vi "QuantelDataGrab.vi"(9 "stop":bool) -> ()   [LabVIEW 2022 SP3]
uses:
  ScanningControl/Pulsers/pulser.ctl
  ScanningControl/Pulsers/UTEX/Controls/UTEX Controls.ctl
  <vilib>/Utility/miscctls.llb/LVRectTypeDef.ctl
  <vilib>/Utility/miscctls.llb/LVBoundsTypeDef.ctl
  ScanningControl/Motion Controllers/NI_controller/-NI_MotionRoutines/MotionParameters.ctl
  ScanningControl/Motion Controllers/NI_controller/-NI_MotionRoutines/MotionSys.ctl
  ScanningControl/Motion Controllers/-MotionRoutines/ScanAxis.ctl
  ScanningControl/Motion Controllers/-MotionRoutines/3rdAxis.ctl
  <vilib>/Utility/miscctls.llb/LVCursorListTypeDef.ctl
  ScanningControl/-ScanSystem/Controls/location.ctl
  ScanningControl/Digitizers/-DigitizerRoutines/Digitizer.ctl
  <vilib>/picture/picture.llb/imagedata.ctl
  <vilib>/Platform/TimedLoop/XDataNode/timing_clust.ctl
  <vilib>/Platform/TimedLoop/XDataNode/nitl_modes.ctl
  <vilib>/Platform/TimedLoop/XDataNode/wakeup.ctl
  <vilib>/event_ctls.llb/eventvkey.ctl
  <vilib>/DAQmx/write.llb/DAQmx Write (Digital Bool 1Line 1Point).vi
  <vilib>/Utility/error.llb/Trim Whitespace One-Sided.vi
  ScanningControl/Pulsers/PulserGlobals.vi
  ScanningControl/Digitizers/-DigitizerRoutines/DigitizerGlobals.vi
  ScanningControl/Motion Controllers/-MotionRoutines/MotionGlobals.vi
  <vilib>/DAQmx/miscellaneous.llb/DAQmx Fill In Error Info.vi
  C:/Windows/System32/ADQAPI_dotNet_helper.dll
  Windows/System32/ADQAPI_dotNet_helper.dll
  <vilib>/Platform/TimedLoop/XDataNode/XDataNode.xnode
  <instrlib>/Acqiris Bx/Acqiris Bx.lvlib
  <instrlib>/LeCroy Wave Series/LeCroy Wave Series.lvlib
  <vilib>/ptbypt/NI_PtbyPt.lvlib
  <instrlib>/Acqiris Dx/Acqiris Dx.lvlib
  <vilib>/Platform/TimedLoop/XDataNode/XDNodeRunTimeDep.lvlib
panel:
  out "Raw data":dbl[][](graph)
  in  "Overide Gain?":bool
  in  "Sector?":bool=TRUE
  in  "Fill\nSpace":bool
  out "File Name":string="none"
  in  "1:1\nAspect":bool
  out "append letter":i8=65
  in  "Visible":bool
  in  "Center":bool
  in  "c (m/s)":dbl=1485.0
  in  "Tab Control":enum32{"Acquire", "Custom Settings", "Pulser"}(tab)
  in  "Scan Location":enum32{"Radio Selection 1", "Radio Selection 2"}(radio)
  in  "View Queue":bool
  out "No data\nEntering\nQueue":bool
  in  "Probe":u16(ring) items=["50MHz", "80MHz", "Custom"]
  out "fps":dbl format="%#.2g"
  in  "Save All Queue":bool
  in  "Flush Queue":bool
  in  "Save Raw":bool
  in  "Pause":bool=TRUE
  out "In Queue":u8 max=50 step=1
  in  "Plane":i8(knob)=1 min=1 max=12 step=1 scale=0.0..4.0
  in  "Gain":dbl(ring)=0.2 items=["7"=8.0, "6"=4.0, "5"=2.0, "4"=0.8, "3"=0.4, "2"=0.2, "1"=0.08]
  in  "Acquire Data":bool
  in  "Name add on":u16(ring) items=["", "_POC_Data_Singapore", "_QUS", "_PE"]
  in  "Patient Info":bool
  in  "SavePath":path=path "C:/POC_Data_Singapore"
  in  "SetDig":bool
  in  "Gate Length":dbl=0.15 format="%.6f"
  in  "LowTime":dbl=0.0001
  in  "Filter Prams":T1={"low cutoff"=20, "order"=81, "high cutoff"=60}
  in  "Type of Mean":u16(ring)=4 items=["Mean from lines", "Mean just lines", "Poly Mean", "No mean", "Filter"]
  in  "distance?":bool=TRUE
  in  "Scan Info":T2
  in  "Timeout (s)":dbl=0.15
  in  "Software Gate":bool=TRUE
  in  "Bang Trig":bool=TRUE
  in  "N to save":u16=100 min=1 max=200 step=1
  out "Current Image":i32
  in  "Save Setting Profile":bool
  in  "Acq Params":T3={"Sampling Rate"=250.0, "Ref Delay (ms)"=0.0, "rf points per line"=2048, "rf lines"=256, "Dig Scale"=4.0} {"Dig Scale" items=["8 V"=8.0, "4 V"=4.0, "2 V"=2.0, "800 mV"=0.8, "400 mV"=0.4, "200 mV"=0.2, "80 mV"=0.08]; "rf lines" min=1; "rf points per line" min=1; "Ref Delay (ms)" format="%.2f"}
  in  "Pulser":T4=enum."UTEX"
  in  "UT340 Controls":T5={"High Pass On"=FALSE, "High Pass Filter (MHz)"=1, "Low Pass On"=FALSE, "Low Pass Filter (MHz)"=20, "PE Gain (dB)"=1, "Voltage"=100, "Pulse Width (ns)"=2.0, "Mode"=FALSE, "PC Gain (dB)"=1, "Trig Source"=FALSE, "Rep Rate (Hz)"=0, "PULSE"=FALSE} {"Low Pass Filter (MHz)" min=20 step=1; "High Pass Filter (MHz)" min=1 max=20 step=1; "Pulse Width (ns)" min=2.0 max=71.75; "Voltage" min=100 max=250 step=2; "PC Gain (dB)" min=0 max=63 step=1; "PE Gain (dB)" min=-6 max=57 step=1}
  in  "dB Range":cluster{i32, i32}(slide)={-65, 0}
  # "dB"
  # "Ruler"
  # "© 2021-22 Weill Cornell"
  # "Do not adjust!!!!!"
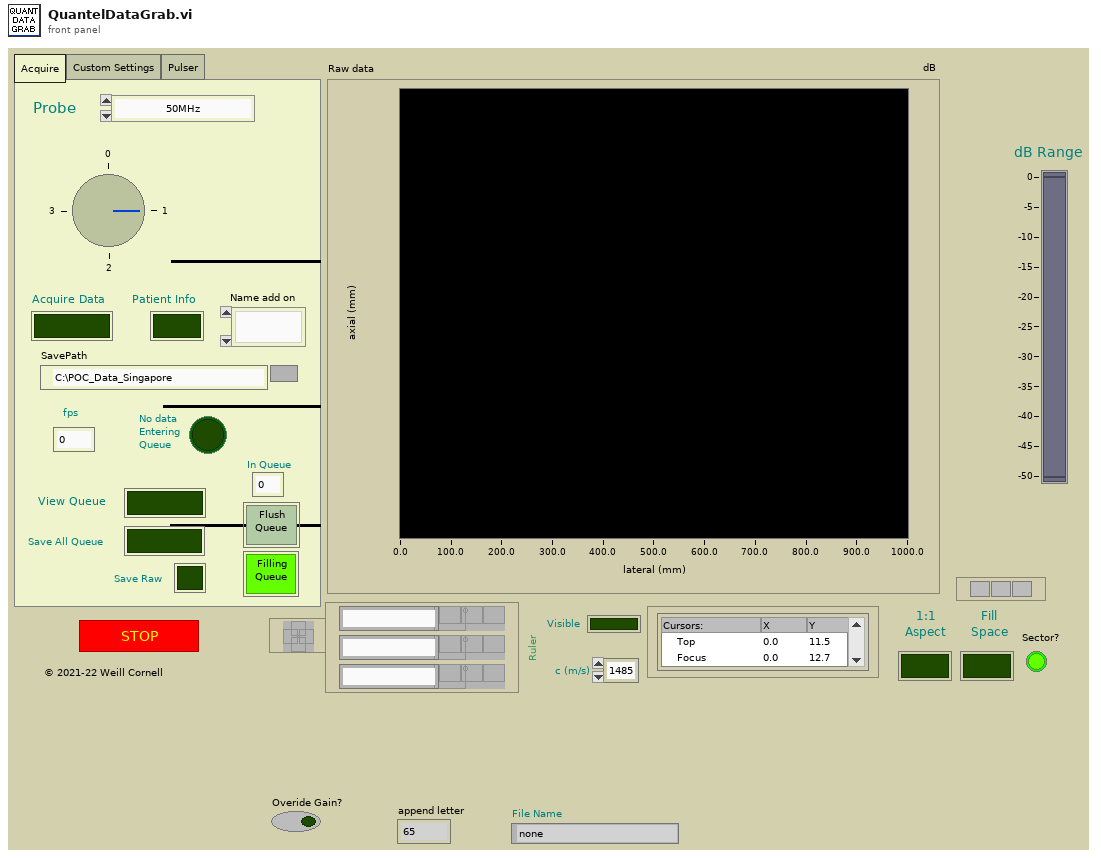
[diagram p1: front panel]
types:
  T1 = cluster{"low cutoff":i32, "order":i32, "high cutoff":i32}
  T2 = cluster{"delay":sgl, "pivot distance":sgl, "sector scan angle":sgl, "operator":string, "Scan Mode":string, "location":string}
  T3 = cluster{"Sampling Rate":dbl, "Ref Delay (ms)":dbl, "rf points per line":i32, "rf lines":i32, "Dig Scale":dbl}
  T4 = typedef "pulser.ctl" = enum16{"Pan 5900", "Daxsonics", "Agilent 33xxx", "UTEX", "JSR", "WMC Mono-Cycle", "No Pulser", "NYU AVTECH", "Tabor W1281A", "Pan 5800", "Unlisted", "Tabor WX2182B"}
  T5 = typedef "UTEX Controls.ctl" = cluster{"High Pass On":bool, "High Pass Filter (MHz)":i16, "Low Pass On":bool, "Low Pass Filter (MHz)":i16, "PE Gain (dB)":i16, "Voltage":i16, "Pulse Width (ns)":dbl, "Mode":bool, "PC Gain (dB)":i16, "Trig Source":bool, "Rep Rate (Hz)":i16, "PULSE":bool}
  T6 = typedef "LVCursorListTypeDef.ctl" = cluster{"Name":string, "Color":u32, "Style":u8, "Point Style":u8, "Name Visible":bool, "Allow Drag":bool, "Cursor Mode":u32, "Plot":i32, "Index":i32, "Position":cluster{"X":dbl, "Y":dbl}, "X Scale":u32, "Y Scale":u32, "Watch Plots":i32[], "Watch All Plots":bool, "Plot Area":i32, "Label Offset":cluster{"X":dbl, "Y":dbl}}[]
  T7 = cluster{"NI Dig":refnum<k15>, "Lecroy":refnum<visa-resource-name>, "Alazar":i32, "Acqiris":string}
  T8 = typedef "MotionParameters.ctl" = cluster{"No Motion?":bool, "Motion System":T9, "Motion Bd ID":u8, "Motion Profile":string, "# Axis":i8, "Reverse Z axis?":bool, "SMAC Axis":u16, "scan pair":T10, "RT fps":sgl, "Steps per mm":i32[], "Motor Parameters":cluster{"velocity ct/s":dbl[], "accel ct/s^2":dbl[]}, "One Way Scan":bool, "Reverse One Way Scan":bool, "Global Position (mm)":dbl[], "Plane":i32, "Distance between\nscan lines (um)":sgl, "Distance between\nscan planes (um)":sgl, "number of scan planes":i32, "Total steps in line":i32, "Xtra plane\ndistance  (um)":i32, "Xtra planes ":i32, "Add Axis":bool, "overshoot cts":i32, "BKPT Shift":i32, "Scan Start Time (ms)":u32, "ESP VISA":refnum<visa-resource-name>, "3rd Axis":T11, "GL Ref Out":refnum<k7>, "Galil Address":string}
  T9 = typedef "MotionSys.ctl" = enum16{"MM3000", "NI 735x", "Newport ESP", "No Motion Card", "Galil"}
  T10 = typedef "ScanAxis.ctl" = enum16{"y-(x) scan", "x-(y) scan", "z-(x) scan", "z-(y) scan", "y-(z) scan", "x-(z) scan", "w-(x) scan", "w-(y) scan", "w-(z) scan", "x-(w) scan", "y-(w) scan", "z-(w) scan"}
  T11 = typedef "3rdAxis.ctl" = u16
  T12 = typedef "LVBoundsTypeDef.ctl" = cluster{"Width":u32, "Height":u32}
  T13 = typedef "LVRectTypeDef.ctl" = cluster{"Left":i16, "Top":i16, "Right":i16, "Bottom":i16}
  T14 = typedef "location.ctl" = enum16{"Automatic", "WCM Main", "Hawaii", "Columbia MM3000", "Columbia  NI System", "NYU", "RRI 2", "UHI Allen", "CUMC RT", "Chiba", "Stony Brook", "WCM Microscopy", "WCM Aeoretch", "WCM Optics Lab", "WCM Main 2Axis", "WCM Rotation", "WCM SAM SMAC", "SERI GP"}
  T15 = typedef "Digitizer.ctl" = enum16{"Acqiris Digitizer", "NI Digitizer", "LeCroy", "GaGe", "AlazarTech", "No Digitizer", "Teledyne"}
  T16 = cluster{"gain":dbl, bool, "wfm":i16[][], "max queue size (-1, unlimited)":i32, bool}
  T17 = cluster{"DataBufferQ":refnum<queue>, "LastNQ":refnum<queue>, "LastN_JPG_Q":refnum<queue>, "Stop":refnum<notifier>}
  T18 = typedef "imagedata.ctl" = cluster{"image type":i32, "image depth":i32, "image":u8[], "mask":u8[], "colors":u32[], "Rectangle":cluster{"left":i16, "top":i16, "right":i16, "bottom":i16}}
  T19 = cluster{"Voltage Scale":dbl, "Offset":dbl, "Coupling":u16}
  T20 = cluster{"Source":u16, "Coupling":u16, "Slope":u16, "Level":dbl}
  T21 = cluster{"Source":u16, "Coupling":u16, "Slope":u16, "Level (mV)":dbl}
  T22 = cluster{"DataBufferQ":refnum<queue>, "LastNQ":refnum<queue>, "LastNBMPQ":refnum<queue>, "SaveRawN":refnum<notifier>, "StopN":refnum<notifier>}
  T23 = cluster{"Active Cursor":u32, "Cursor.Cursor Color":u32, "Cursor.Cursor Position:Cursor Y":dbl, "Cursor.Cursor Position:Cursor X":dbl, "Cursor.Cursor Style":u8, "Cursor.Line Style":u8, "Cursor.Line Width":u8, "Cursor.Visible":bool}[]
  T24 = typedef "XDNodeRunTimeDep.lvlib/timing_clust.ctl" = cluster{"Expected End [f-1]":u64, "Actual End [f-1]":u64, "Finished Late? [f-1]":bool, "Expected End [i-1]":u64, "Actual End [i-1]":u64, "Finished Late? [i-1]":bool, "Expected Start [i]":u64, "Actual Start [i]":u64, "Expected Start [f]":u64, "Actual Start [f]":u64, "Source Name":string, "Structure Name":string, "Period":i64, "Deadline":i64, "Offset":i64, "Start":i64, "Priority":i32, "Timeout":i32, "Mode":T25, "Wakeup Reason":T26, "Error":errorcluster, "Source Type":string, "Secondary Source Type":string, "Global End Time":u64, "Global Start Time":u64, "Frame Duration":u64, "Iteration Duration":u64, "Assigned CPU":i32, "I/O Scan Engine Mode":u32}
  T25 = typedef "XDNodeRunTimeDep.lvlib/nitl_modes.ctl" = enum32{"No Change", "Process missed periods, maintain original phase", "Discard missed periods, maintain original phase", "Process missed periods, ignore original phase", "Discard missed periods, ignore original phase"}
  T26 = typedef "XDNodeRunTimeDep.lvlib/wakeup.ctl" = enum32{"Normal", "Aborted", "Asynchronous wakeup", "Timing source error", "Timed loop error", "Timeout"}
  T27 = typedef "eventvkey.ctl" = enum16{"ASCII", "Enter", "Return", "Shift", "Ctrl", "Alt", "Cmd", "Opt", "Caps", "NumLock", "Clear", "Break", "Up", "Down", "Left", "Right", "Insert", "Delete", "Home", "End", "PageUp", "PageDown", "Escape", "Help", "Pause", "ScrollLock", "F1", "F2", "F3", "F4", "F5", "F6", "F7", "F8", "F9", "F10", "F11", "F12", "F13", "F14", "F15", "F16", "F17", "F18", "F19", "F20", "F21", "F22", "F23", "F24", "Play", "VolumeUp", "VolumeDown", "Mute", "Two Byte Char"}
  T28 = typedef "DigitizerSettings.ctl" = cluster{"Digitizer delay (us) ":dbl, "rf points per line":i32, "lines per plane":i32, "Samp Rate (Hz)":dbl, "Additional dig delay (us)":dbl, "Voltage Scale":dbl, "Pre-Looks":i32, "Offset delay (us)":dbl, "bits A/D":i8, "Avg Num":i32, "DigTimeOut":sgl, "Rel Dig Delay":sgl, "Dig Ch":i32, "LeCroyCluster":cluster{"LeCroy Channels":bool[], "LC read pt offset":dbl, "Sweep Avg":bool}, "Main Digitizer":T15, "Dig Config":T29, "Digitizer ID Cluster":T30, "Trigger Settings":cluster{"Trig Source":u16, "Trig Coupling":u16, "Trig Slope":u16, "Level (mV)":dbl}, "Bulk Acq":bool, "Bulk Start Indexes":i32[], "Data Ref RF":refnum<data-value>, "NI ID/Channel":cluster{"NI ID":refnum<k15>, "NI CH":i32}[], "Total Dig CH":i32, "Xtra Ann Trig delay (us)":dbl, "Fix Z Delay?":bool, "One Way Transmission?":bool, "Data Ref Log":refnum<data-value>}
  T29 = typedef "DigConfig.ctl" = enum16{"Single channel", "2 Chans w/ 2 Acqiris", "2 Chans w/ 1 Acqiris", "5-CH Pulser New", "5-CH pulser w/ ann array", "5-pass style ann array", "Empty"}
  T30 = typedef "DigitizerID.ctl" = cluster{"Acqiris/Alazar/SP ID":u32[], "NI Instr Handles":refnum<k15>[], "LeCroy VISA":refnum<visa-resource-name>, "GaGe Handle":cluster{"Handle":u32, "Sample size":u32, "Resolution":i32, "Offset":i32, "Channels":u32, "Boards":u32}, "ATS Ref":string, "Acqiris Address":string[], "ADQRef":refnum<k24>, "adq_cu_ptr":refnum<k24>}
  T31 = cluster{"Handle":u32, "Sample size":u32, "Resolution":i32, "Offset":i32, "Channels":u32, "Boards":u32}
  T32 = typedef "LVStringsAndValuesArrayTypeDef_DBL.ctl" = cluster{"String":string, "Value":dbl}[]
  T33 = cluster{"Case name":string, "Distance between\nscan lines (mm)":sgl, "Acquistion Parameters":cluster{"Sampling Rate":dbl, "Ref Delay (ms)":dbl, "rf points per line":i32, "rf lines":i32, "Dig Scale":dbl}, "Timeout (s)":dbl, "Sector?":bool, "Filter Prams":cluster{"low cutoff":i32, "order":i32, "high cutoff":i32}, "Scan Info":cluster{"delay":sgl, "pivot distance":sgl, "sector scan angle":sgl, "operator":string, "Scan Mode":string, "location":string}, "UT340 Controls":T5}[]
  T34 = cluster{"Case name":string, "Distance between\nscan lines (mm)":sgl, "Acquistion Parameters":cluster{"Sampling Rate":dbl, "Ref Delay (ms)":dbl, "rf points per line":i32, "rf lines":i32, "Dig Scale":dbl}, "Timeout (s)":dbl, "Sector?":bool, "Filter Prams":cluster{"low cutoff":i32, "order":i32, "high cutoff":i32}, "Scan Info":cluster{"delay":sgl, "pivot distance":sgl, "sector scan angle":sgl, "operator":string, "Scan Mode":string, "location":string}, "UT340 Controls":T5}
  T35 = cluster{"data value reference":refnum<data-value>, "bytes to transfer":u32, "rf pts actual":u32}
  T36 = cluster{"Y Scale Offset":dbl, "Y Scale Multi":dbl, "X Scale Offset":dbl, "X Scale Multi":dbl, "Gate Distance":dbl}
  T37 = cluster{"Axis scaling Params":cluster{"X right":dbl, "X left":dbl, "Y low":dbl, "Y high":dbl}, "x scaled":dbl[][], "y scaled":dbl[][], "scales":cluster{"inc x (mm)":dbl, "inc y (mm)":dbl}, "Array":dbl[][], "pixels in x":i16, "pixels in y":i16}
  T38 = cluster{"Sampling Rate":dbl, "Ref Delay (ms)":dbl, "rf points per line":i32}
  T39 = cluster{"Sampling Rate":dbl, "Ref Delay (ms)":dbl, "rf points per line":i32, "lines per plane":i32, "Voltage Scale":dbl}
  T40 = typedef "PatientInfoDef.ctl" = cluster{"Eye Selector":enum32{"Left", "Right"}, "Plane":i8, "First Name":string, "Last Name":string, "Notes":string, "Patient ID":string, "Scan Location":enum32{"Radio Selection 1", "Radio Selection 2"}}
  T41 = typedef "LVRangeTypeDef.ctl" = cluster{"Minimum":dbl, "Maximum":dbl, "Increment":dbl, "Minor Increment":dbl, "Start":dbl}
  T42 = typedef "LVPointDoubleTypeDef.ctl" = cluster{"Cursor X":dbl, "Cursor Y":dbl}
  T43 = cluster{"New Case Name":string, "Distance between\nscan lines (um)":sgl, "Acq Params":cluster{"Sampling Rate":dbl, "Ref Delay (ms)":dbl, "rf points per line":i32, "rf lines":i32, "Dig Scale":dbl}, "Timeout (s)":dbl, "Sector?":bool, "Filter Prams":cluster{"low cutoff":i32, "order":i32, "high cutoff":i32}, "Scan Info":cluster{"delay":sgl, "pivot distance":sgl, "sector scan angle":sgl, "operator":string, "Scan Mode":string, "location":string}, "Value":T5}
  T44 = cluster{"High Pass On":bool, "High Pass Filter (MHz)":bool, "Low Pass On":bool, "Low Pass Filter (MHz)":bool, "PE Gain (dB)":bool, "Voltage":bool, "Pulse Width (ns)":bool, "Mode":bool, "PC Gain (dB)":bool, "Trig Source":bool, "Rep Rate (Hz)":bool, "PULSE":bool}
  T45 = cluster{"gain":dbl, "status":bool, "Array":i16[][], "timeout in ms (-1)":i32, "status":bool}
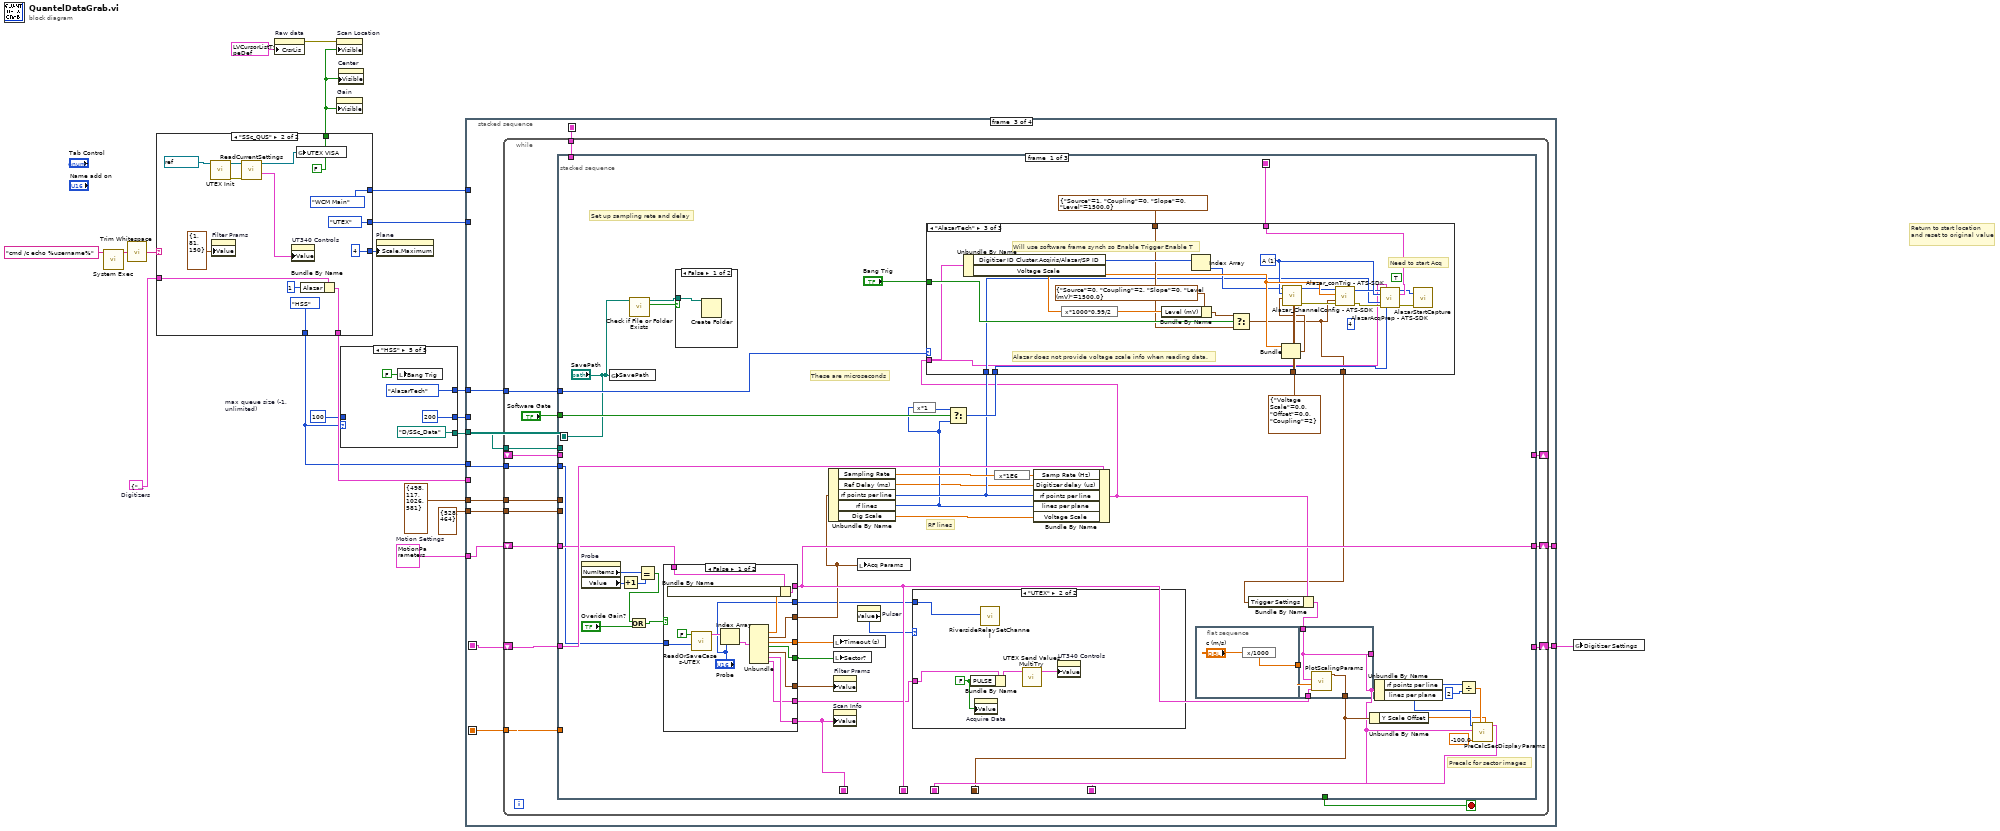
[diagram p0: block diagram]
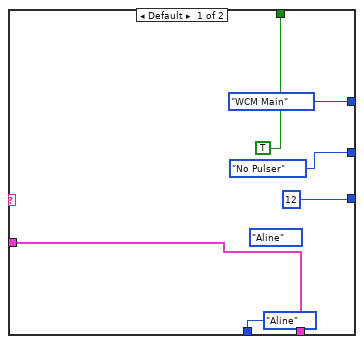
[diagram p2: hidden frame]
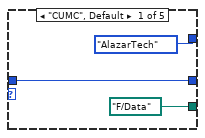
[diagram p3: hidden frame]
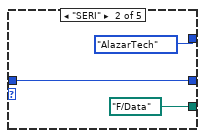
[diagram p4: hidden frame]
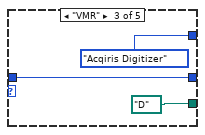
[diagram p5: hidden frame]
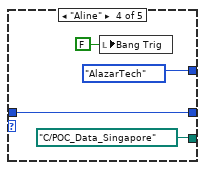
[diagram p6: hidden frame]
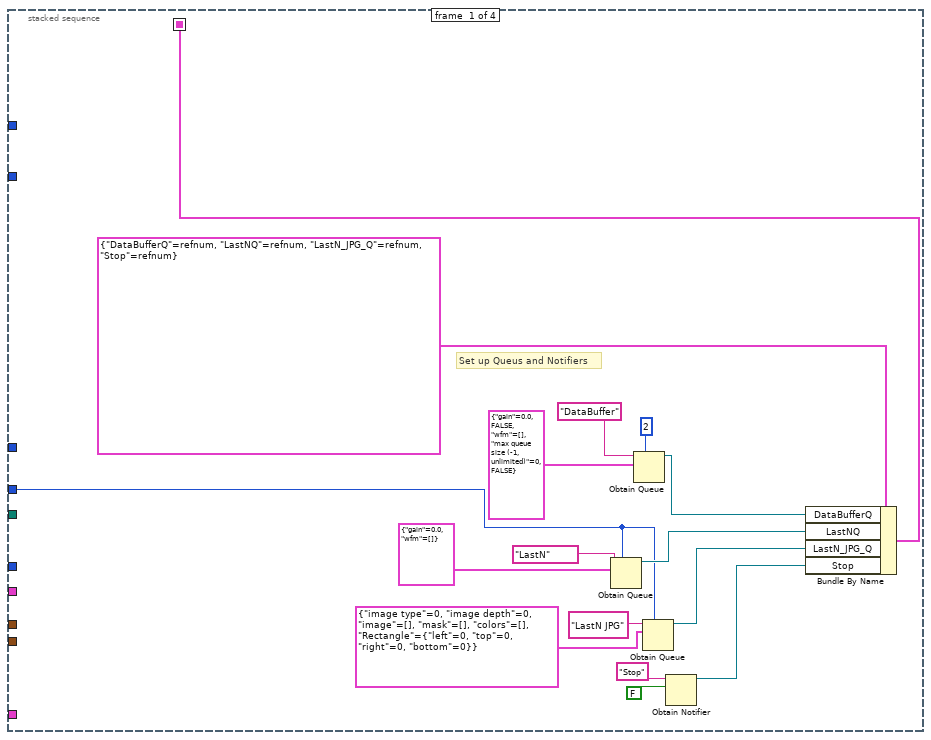
[diagram p7: hidden frame]
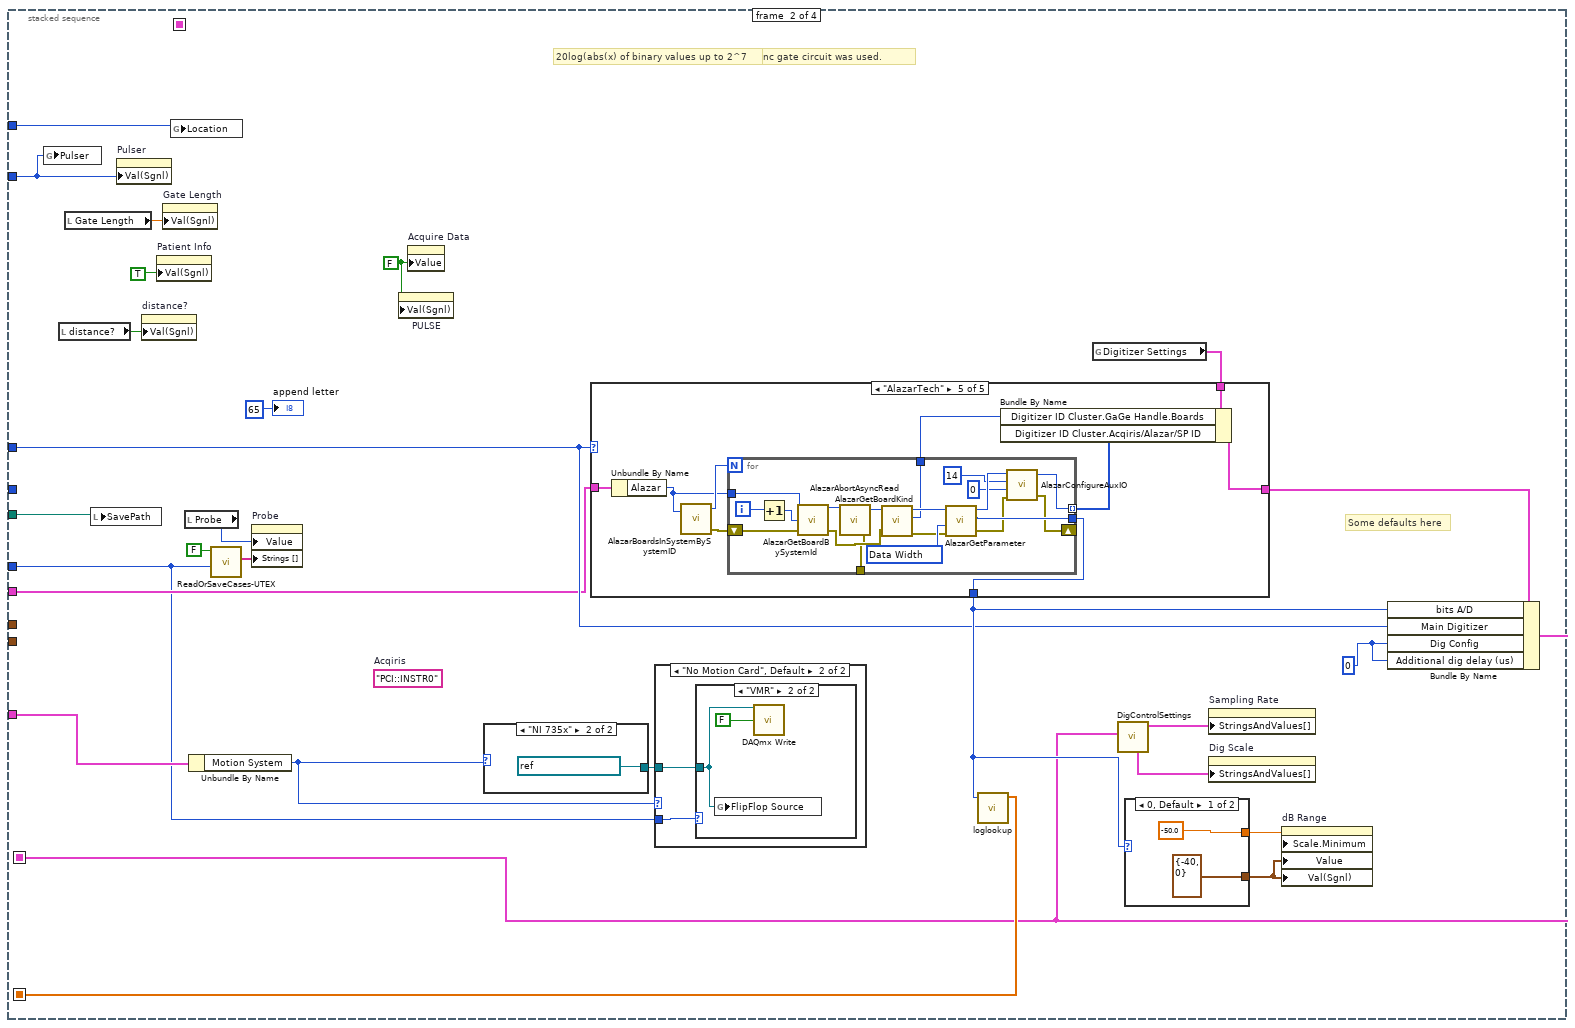
[diagram p8: hidden frame]
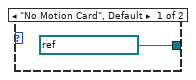
[diagram p11: hidden frame]
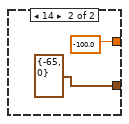
[diagram p12: hidden frame]
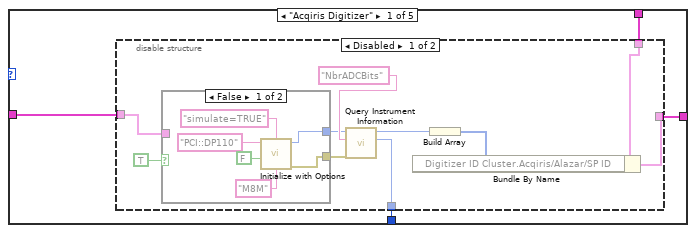
[diagram p13: hidden frame]
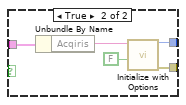
[diagram p14: hidden frame]
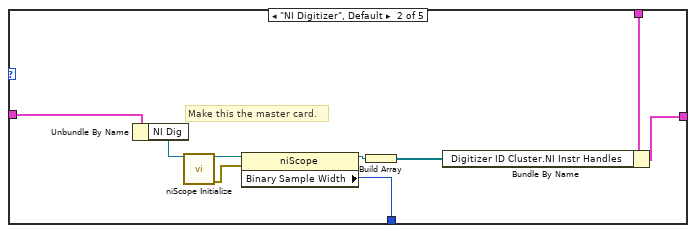
[diagram p16: hidden frame]
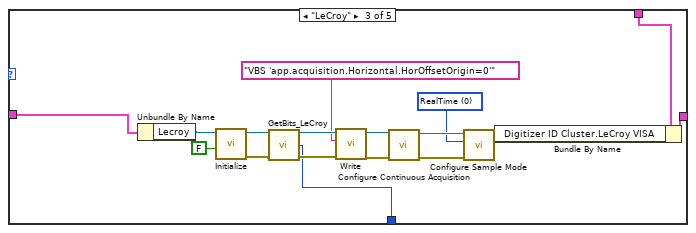
[diagram p17: hidden frame]
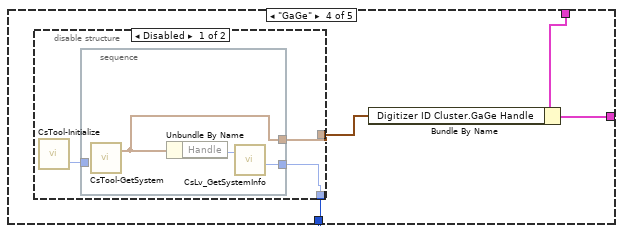
[diagram p18: hidden frame]
diagram:
  w5 = 100  # max queue size (-1, unlimited)
  w10 = T7 {"NI Dig"="Dig1", "Lecroy"="VICP::169.254.51.39", "Alazar"=0, "Acqiris"="PCI::SER10157"}  # Digitizers
  w18 = T8 {"No Motion?"=FALSE, "Motion System"=enum."No Motion Card", "Motion Bd ID"=1, "Motion Profile"="SMAC1", "# Axis"=1, "Reverse Z axis?"=TRUE, "SMAC Axis"=0, "scan pair"=enum."y-(x) scan", "RT fps"=6.0, "Steps per mm"=[1000, 1000, 1000, 1000], "Motor Parameters"={"velocity ct/s"=[10000.0, 10000.0, 10000.0, 50000.0], "accel ct/s^2"=[50000.0, 50000.0, 50000.0, 200000.0]}, "One Way Scan"=FALSE, "Reverse One Way Scan"=FALSE, "Global Position (mm)"=[], "Plane"=0, "Distance between\nscan lines (um)"=0.0, "Distance between\nscan planes (um)"=0.0, "number of scan planes"=1, "Total steps in line"=0, "Xtra plane\ndistance  (um)"=100, "Xtra planes "=1, "Add Axis"=FALSE, "overshoot cts"=200, "BKPT Shift"=0, "Scan Start Time (ms)"=0, "ESP VISA"="GPIB::1::INSTR", "3rd Axis"=1, "GL Ref Out"=refnum, "Galil Address"=""}  # Motion Settings
  # "Return to start location and reset to original value"
  n1 = call <vilib>:"System Exec.vi"("command line"="cmd /c echo %username%") -> ("standard output"=w13:string)  [unwired: 7 in, 3 out]
  n2 = call <vilib>:"Trim Whitespace.vi"("string"=w13) -> ("trimmed string"=w12:string)  [unwired: 1 in]
  n3 = case shown="\"SSc_QUS\"" w12 {
    tunnel: [TRUE FALSE] -> w1
    tunnel: [12 4] -> w11
    tunnel: [w24 w37] -> w9
    tunnel: w10 -> [w24 w38]
    tunnel: [pulser."No Pulser" ("Pulser") pulser."UTEX" ("Pulser")] -> w8
    tunnel: [location."WCM Main" ("Location") location."WCM Main" ("Location")] -> w7
    tunnel: [enum16{"CUMC", "SERI", "VMR", "Aline", "HSS"}."Aline" ("Location") enum16{"CUMC", "SERI", "VMR", "Aline", "HSS"}."HSS" ("Location")] -> w6
    frame Default {
      (unwired) enum16{"CUMC", "SERI", "VMR", "Aline", "UTEX"}."Aline"
    }
    frame "SSc_QUS" {
      n4 = call "UTEX Init.vi"("VISA resource name"=refnum<visa-resource-name> "UTEX" ("UTEX VISA")) -> ("error out"=w32:errorcluster, "VISA resource Out"=w30:refnum<visa-resource-name>)  [unwired: 9 in]
      n5 = property on="Filter Prams" class="Clust (strict)"("Value"=T1 {"low cutoff"=1, "order"=81, "high cutoff"=150} ("Filter Prams")) -> ()  [unwired: 2 in, 2 out]
      n6 = call "ReadCurrentSettings.vi"("error in (no error)"=w32, "VISA Refnum in"=w30) -> ("UT340 Controls"=w29:T5, "VISA Refnum out"=w28:refnum<visa-resource-name>)  [unwired: 7 in, 1 out]
      n7 = property on="UT340 Controls" class="Clust (strict)"("Value"=w29) -> ()  [unwired: 2 in, 2 out]
      n8 = global write "PulserGlobals.vi" "UTEX VISA"(w28) -> ()
      n9 = Bundle By Name(cluster=w38, "Alazar"=1) -> (w37:T7)
    }
  }
  n10 = property on="Raw data" class="IntGraph (strict)"("CrsrLis"=T6 [{"Name"="Top", "Color"=0, "Style"=0, "Point Style"=0, "Name Visible"=FALSE, "Allow Drag"=FALSE, "Cursor Mode"=0, "Plot"=0, "Index"=0, "Position"={"X"=0.0, "Y"=0.0}, "X Scale"=0, "Y Scale"=0, "Watch Plots"=[], "Watch All Plots"=FALSE, "Plot Area"=0, "Label Offset"={"X"=0.0, "Y"=0.0}}, {"Name"="Focus", "Color"=0, "Style"=0, "Point Style"=0, "Name Visible"=FALSE, "Allow Drag"=FALSE, "Cursor Mode"=0, "Plot"=0, "Index"=0, "Position"={"X"=0.0, "Y"=0.0}, "X Scale"=0, "Y Scale"=0, "Watch Plots"=[], "Watch All Plots"=FALSE, "Plot Area"=0, "Label Offset"={"X"=0.0, "Y"=0.0}}] ("Cursor List")) -> (error out=w2:errorcluster)  [unwired: 2 in, 1 out]
  n11 = property on="Scan Location" class="RadioBtnsControl (strict)"(error in=w2, "Visible"=w1) -> ()  [unwired: 1 in, 2 out]
  n12 = property on="Gain" class="Ring (strict)"("Visible"=w1) -> ()  [unwired: 2 in, 2 out]
  n13 = property on="Center" class="Bool"("Visible"=w1) -> ()  [unwired: 2 in, 2 out]
  n14 = case shown="\"HSS\"" w6 {
    tunnel: [path "F:/Data" ("SavePath") path "F:/Data" ("SavePath") path "D:/" ("SavePath") path "C:/POC_Data_Singapore" ("SavePath") path "D:/SSc_Data" ("SavePath")] -> w20
    tunnel: [Digitizer."AlazarTech" ("Main Digitizer") Digitizer."AlazarTech" ("Main Digitizer") Digitizer."Acqiris Digitizer" ("Main Digitizer") Digitizer."AlazarTech" ("Main Digitizer") Digitizer."AlazarTech" ("Main Digitizer")] -> w19
    tunnel: [w41 w44 w47 w50 200 ("max queue size (-1, unlimited)")] -> w4
    tunnel: w5 -> [w41 w44 w47 w50 _]
    frame "CUMC", Default {
    }
    frame "SERI" {
    }
    frame "VMR" {
    }
    frame "Aline" {
      n15 = local write "Bang Trig"(FALSE ("Bang Trig")) -> ()
    }
    frame "HSS" {
      n16 = local write "Bang Trig"(FALSE ("Bang Trig")) -> ()
    }
  }
  n17 = property on="Plane" class="Knob (strict)"("Scale.Maximum"=w11) -> ()  [unwired: 2 in, 2 out]
  n18 = stacked-sequence {
    seq-local: [_ w100 _ _] -> [_ _ w210 _]
    seq-local: [w63 _ _ _] -> [_ _ w208 w957]
    seq-local: [_ w82 _ _] -> [_ _ w202 w956]
    tunnel: w19 -> [_ w81 w209 _]
    tunnel: T12 {"Width"=528, "Height"=464} ("Plot Area:Size") -> [_ _ w207 _]
    tunnel: T13 {"Left"=498, "Top"=117, "Right"=1026, "Bottom"=581} ("Plot Area Bounds") -> [_ _ w206 _]
    tunnel: w20 -> [_ w80 w205 _]
    tunnel: w6 -> [_ w76 w204 _]
    tunnel: [_ _ w203 _] -> w17
    tunnel: w18 -> [_ w87 w201 _]
    tunnel: [_ _ w200 _] -> _
    tunnel: w9 -> [_ w78 _ _]
    tunnel: w8 -> [_ w75 _ _]
    tunnel: w7 -> [_ w77 _ _]
    tunnel: w4 -> [w58 _ _ _]
    frame #0 {
      # "Set up Queus and Notifiers"
      n19 = Obtain Queue ("LastN")(max queue size (-1, unlimited)=w58, name (unnamed)="LastN", element data type=cluster{"gain":dbl, "wfm":i16[][]} {"gain"=0.0, "wfm"=[]}) -> (queue out=w62:refnum<queue>)  [unwired: 2 in, 2 out]
      n20 = Obtain Queue(max queue size (-1, unlimited)=2, name (unnamed)="DataBuffer", element data type=T16 {"gain"=0.0, FALSE, "wfm"=[], "max queue size (-1, unlimited)"=0, FALSE}) -> (queue out=w59:refnum<queue>)  [unwired: 2 in, 2 out]
      n21 = Obtain Queue ("LastNBMP")(max queue size (-1, unlimited)=w58, name (unnamed)="LastN JPG", element data type=T18 {"image type"=0, "image depth"=0, "image"=[], "mask"=[], "colors"=[], "Rectangle"={"left"=0, "top"=0, "right"=0, "bottom"=0}} ("Image Data")) -> (queue out=w68:refnum<queue>)  [unwired: 2 in, 2 out]
      n22 = Obtain Notifier ("Raw eye")(name (unnamed)="Stop", notification data type=FALSE) -> (notifier out=w64:refnum<notifier>)  [unwired: 2 in, 2 out]
      n23 = Bundle By Name(cluster=T17 {"DataBufferQ"=refnum, "LastNQ"=refnum, "LastN_JPG_Q"=refnum, "Stop"=refnum} ("Qs and Notis"), "DataBufferQ"=w59, "LastNQ"=w62, "LastN_JPG_Q"=w68, "Stop"=w64) -> (w63:T17)
    }
    frame #1 {
      w74 = FALSE ("Acquire Data")
      (unwired) "PCI::INSTR0"  # Acqiris
      w88 = 0 ("Dig Config")
      # "Left Over stuff from when external frame sync gate circuit was used."
      # "Some defaults here"
      # "20log(abs(x) of binary values up to 2^7"
      n24 = global write "PulserGlobals.vi" "Pulser"(w75) -> ()
      n25 = local read "distance?"() -> (w79:bool)
      n26 = local read "Gate Length"() -> (w99:dbl)
      n27 = local write "SavePath"(w80) -> ()
      n28 = property on="Pulser" class="Enum (strict)"("Val(Sgnl)"=w75) -> ()  [unwired: 2 in, 2 out]
      n29 = property on="distance?" class="Bool (strict)"("Val(Sgnl)"=w79) -> ()  [unwired: 2 in, 2 out]
      n30 = property on="Patient Info" class="Bool (strict)"("Val(Sgnl)"=TRUE ("Value (Signaling)")) -> ()  [unwired: 2 in, 2 out]
      n31 = property on="Gate Length" class="DigNum (strict)"("Val(Sgnl)"=w99) -> ()  [unwired: 2 in, 2 out]
      n32 = global write "MotionGlobals.vi" "Location"(w77) -> ()
      n33 = local read "Probe"() -> (w90:u16)
      n34 = Unbundle By Name(w87) -> ("Motion System"=w86:T9)
      n35 = call "ReadOrSaveCases-UTEX.vi"("Location"=w76, "Save(T)\\Read(F)"=FALSE ("Save(T)\\Read(F)")) -> ("Case List"=w91:string[])  [unwired: 8 in, 1 out]
      n36 = property on="Probe" class="Ring (strict)"("Value"=w90, "Strings []"=w91) -> ()  [unwired: 2 in, 2 out]
      n37 = property on="PULSE" class="Bool (strict)"("Val(Sgnl)"=w74) -> ()  [unwired: 2 in, 2 out]
      n38 = property on="Acquire Data" class="Bool (strict)"("Value"=w74) -> ()  [unwired: 2 in, 2 out]
      n39 = case shown="\"NI 735x\"" w86 {
        tunnel: [refnum<k21> "Dev1 FlipFlop" ("FlipFlop Source") refnum<k21> "QuantFlipFlop" ("FlipFlop Source")] -> w85
        frame "No Motion Card", Default {
        }
        frame "NI 735x" {
        }
      }
      n40 = case shown="\"No Motion Card\", Default" w86 {
        tunnel: w85 -> [_ w102]
        tunnel: w76 -> [_ w101]
        frame "NI 735x" {
        }
        frame "No Motion Card", Default {
          n41 = case shown="\"VMR\"" w101 {
            tunnel: w102 -> [_ w103]
            frame "CUMC", Default {
            }
            frame "VMR" {
              n42 = global write "MotionGlobals.vi" "FlipFlop Source"(w103) -> ()
              n43 = call-poly <vilib>:"DAQmx Write.vi"("task/channels in"=w103, "data"=FALSE) -> ()  [unwired: 11 in, 3 out]
            }
          }
        }
      }
      n44 = global read "DigitizerGlobals.vi" "Digitizer Settings"() -> (w83:T28)
      n45 = case shown="\"AlazarTech\"" w81 {
        tunnel: [w114 w144 w146 w165 w174] -> w89
        tunnel: w78 -> [w113 w141 w150 _ w173]
        tunnel: [w112 w137 w147 w163 w175] -> w84
        tunnel: w83 -> [w111 w136 w145 w162 w176]
        frame "Acqiris Digitizer" {
          n46 = disable-structure shown="Disabled" {
            disable-tunnel: [w123 _] -> w114
            disable-tunnel: w113 -> [w122 _]
            disable-tunnel: [w119 _] -> w112
            disable-tunnel: w111 -> [w115 _]
            frame Disabled {
              n47 = case shown="False" TRUE {
                tunnel: w122 -> [_ w134]
                tunnel: [w129 w133] -> w118
                tunnel: [w128 w132] -> w117
                frame False {
                  n48 = call <instrlib>:"Initialize with Options.vi"("Options String (null string)"="simulate=TRUE", "Resource Name (PCI::INSTR0)"="PCI::DP110" ("Simulation Options (null string)"), "Simulation Options (null string)"="M8M" ("Options String (null string)"), "Reset (T: Reset)"=FALSE) -> ("Instrument ID"=w129:u32, "error out"=w128:errorcluster)  [unwired: 2 in, 2 out]
                }
                frame True {
                  n49 = Unbundle By Name(w134) -> ("Acqiris"=w131:string)
                  n50 = call <instrlib>:"Initialize with Options.vi"("Resource Name (PCI::INSTR0)"=w131, "Reset (T: Reset)"=FALSE) -> ("Instrument ID"=w133:u32, "error out"=w132:errorcluster)  [unwired: 4 in, 2 out]
                }
              }
              n51 = call <instrlib>:"Query Instrument Information.vi"("Instrument ID"=w118, "Parameter String"="NbrADCBits", "error in (no error)"=w117) -> ("dup Instrument ID"=w121:u32, "Info Value (I32)"=w123:i32)  [unwired: 1 in, 4 out]
              n52 = Build Array(w121) -> (w120:u32[])
              n53 = Bundle By Name(cluster=w115, "Digitizer ID Cluster.Acqiris/Alazar/SP ID"=w120) -> (w119:T28)
            }
            frame Enabled {
            }
          }
        }
        frame "NI Digitizer", Default {
          # "Make this the master card."
          n54 = Unbundle By Name(w141) -> ("NI Dig"=w140:refnum<k15>)
          n55 = call <instrlib>:"niScope Initialize.vi"("resource name"=w140) -> ("instrument handle"=w143:refnum<k15>, "error out"=w142:errorcluster)  [unwired: 3 in, 10 out]
          n56 = property class="niScope"(reference=w143, error in=w142) -> (reference out=w139:refnum<k15>, "Binary Sample Width"=w144:i32)  [unwired: 1 out]
          n57 = Build Array(w139) -> (w138:refnum<k15>[])
          n58 = Bundle By Name(cluster=w136, "Digitizer ID Cluster.NI Instr Handles"=w138) -> (w137:T28)
        }
        frame "LeCroy" {
          w156 = u16 0 items=["RealTime", "RIS", "Sequence", "Roll", "WaveStream"] ("Sample Mode (0: RealTime)")
          n59 = Unbundle By Name(w150) -> ("Lecroy"=w149:refnum<visa-resource-name>)
          n60 = call <instrlib>:"Initialize.vi"("Reset? (T: Yes)"=FALSE, "VISA resource name"=w149) -> ("error out"=w159:errorcluster, "VISA resource name out"=w160:refnum<visa-resource-name>)  [unwired: 8 in]
          n61 = call "GetBits_LeCroy.vi"("VISA resource name"=w160, "error in (no error)"=w159) -> ("VISA resource name out"=w152:refnum<visa-resource-name>, "Nom_Bits"=w146:i16, "error out"=w153:errorcluster)  [unwired: 11 in]
          n62 = call <instrlib>:"Write.vi"("error in (no error)"=w153, "Write Buffer"="VBS 'app.acquisition.Horizontal.HorOffsetOrigin=0'", "VISA resource name"=w152) -> ("error out"=w154:errorcluster, "VISA resource name out"=w155:refnum<visa-resource-name>)  [unwired: 6 in, 1 out]
          n63 = call <instrlib>:"Configure Continuous Acquisition.vi"("error in (no error)"=w154, "VISA resource name"=w155) -> ("error out"=w158:errorcluster, "VISA resource name out"=w157:refnum<visa-resource-name>)  [unwired: 8 in]
          n64 = call <instrlib>:"Configure Sample Mode.vi"("error in (no error)"=w158, "Sample Mode (0: RealTime)"=w156, "VISA resource name"=w157) -> ("VISA resource name out"=w148:refnum<visa-resource-name>)  [unwired: 7 in, 1 out]
          n65 = Bundle By Name(cluster=w145, "Digitizer ID Cluster.LeCroy VISA"=w148) -> (w147:T28)
        }
        frame "GaGe" {
          n66 = disable-structure shown="Disabled" {
            disable-tunnel: [w166 _] -> w165
            disable-tunnel: [w167 _] -> w164
            frame Disabled {
              n67 = call <userlib>:"CsTool-Initialize.vi"() -> ("Error Code"=w168:i32)  [unwired: 1 out]
              n68 = stacked-sequence {
                tunnel: [w170] -> w166
                tunnel: w168 -> [_]
                tunnel: [w169] -> w167
                frame #0 {
                  n69 = call <userlib>:"CsTool-GetSystem.vi"() -> ("Handle Cluster"=w169:T31)  [unwired: 4 in, 1 out]
                  n70 = Unbundle By Name(w169) -> ("Handle"=w171:u32)
                  n71 = call <userlib>:"CsLv_GetSystemInfo.vi"("Handle"=w171) -> ("Sample Bits"=w170:u32)  [unwired: 6 out]
                }
              }
            }
            frame Enabled {
            }
          }
          n72 = Bundle By Name(cluster=w162, "Digitizer ID Cluster.GaGe Handle"=w164) -> (w163:T28)
        }
        frame "AlazarTech" {
          n73 = Unbundle By Name(w173) -> ("Alazar"=w172:i32)
          n74 = call "AlazarBoardsInSystemBySystemID.vi"("System ID"=w172) -> ("Board Count"=w178:u32, "error out"=w177:errorcluster)  [unwired: 1 in, 1 out]
          n75 = for {
            N: w178 -> [_]
            tunnel: [w185] -> w179 mode=indexing
            shift-right: [w183] -> _
            shift-left: w177 -> [w197]
            tunnel: w172 -> [w194]
            tunnel: [w190] -> w180
            tunnel: [w189] -> w174
            tunnel: [w187] -> _
            i -> [w196]
            w199 = u32 268435465 items=["Data Width"=268435465, "Set/Get Async BuffSize"=268435513, "Set/Get Async Buffcount"=268435520, "Get Data Format"=268435522, "Get Samples Per Timestamp Clock"=268435524, "Get Records Captured"=268435525, "Get Async Buffers Pending"=268435536, "Get Async Buffers Pending Full"=268435537, "Get Async Buffers Pending Empty"=268435538, "ECC Mode"=268435528, "Get Aux Input Level"=268435529, "Get Channels Per Board"=268435568, "Pack Mode"=268435570, "Get FPGA Temperature"=268435584] ("Parameter")
            n76 = Increment(x=w196) -> (x+1=w195:i32)
            n77 = call "AlazarGetBoardBySystemId.vi"("error in (no error)"=w197, "Board ID"=w195, "System ID"=w194) -> ("error out"=w188:errorcluster, "Handle"=w198:u64)  [unwired: 1 out]
            n78 = call "AlazarAbortAsyncRead.vi"("Handle"=w198) -> ("Handle"=w193:u64, "error out"=w187:errorcluster)  [unwired: 1 in, 1 out]
            n79 = call "AlazarGetBoardKind.vi"("Handle"=w193, "error in (no error)"=w188) -> ("Handle"=w191:u64, "Board Kind"=w190:u32, "error out"=w192:errorcluster)  [unwired: 1 out]
            n80 = call "AlazarGetParameter.vi"("error in (no error)"=w192, "Parameter"=w199, "Handle"=w191) -> ("error out"=w184:errorcluster, "Value"=w189:i32, "Handle"=w186:u64)  [unwired: 1 in, 1 out]
            n81 = call "AlazarConfigureAuxIO.vi"("error in (no error)"=w184, "Parameter"=u32 0, "Mode"=u32 14, "Handle"=w186) -> ("error out"=w183:errorcluster, "Handle"=w185:u64)  [unwired: 1 out]
          }
          n82 = Bundle By Name(cluster=w176, "Digitizer ID Cluster.GaGe Handle.Boards"=w180, "Digitizer ID Cluster.Acqiris/Alazar/SP ID"=w179) -> (w175:T28)
        }
      }
      n83 = call "loglookup.vi"("A/D bits"=w89) -> ("Log Lookup"=w100:sgl[])  [unwired: 2 in, 3 out]
      n84 = case shown="0, Default" w89 {
        tunnel: [-50.0 ("Scale.Range:Maximum") -100.0 ("Scale.Range:Maximum")] -> w94
        tunnel: [cluster{i32, i32} {-40, 0} ("dB Range") cluster{i32, i32} {-65, 0} ("dB Range")] -> w93
        frame 0, Default {
        }
        frame 14 {
        }
      }
      n85 = property on="dB Range" class="Slide (strict)"("Scale.Minimum"=w94, "Value"=w93, "Val(Sgnl)"=w93) -> ()  [unwired: 2 in, 2 out]
      n86 = Bundle By Name(cluster=w84, "bits A/D"=w89, "Main Digitizer"=w81, "Dig Config"=w88, "Additional dig delay (us)"=w88) -> (w82:T28)
      n87 = call "DigControlSettings.vi"("Digitizer Settings"=w82) -> ("Sampling Rates"=w96:T32, "Voltage Scale"=w95:T32)  [unwired: 6 in, 3 out]
      n88 = property on="Sampling Rate" class="Ring (strict)"("StringsAndValues[]"=w96) -> ()  [unwired: 2 in, 2 out]
      n89 = property on="Dig Scale" class="Ring (strict)"("StringsAndValues[]"=w95) -> ()  [unwired: 2 in, 2 out]
      "append letter" <- i8 65 ("append letter")
    }
    frame #2 {
      n90 = while {
        tunnel: w210 -> [w225]
        tunnel: w209 -> [w223]
        tunnel: w208 -> [w218]
        tunnel: w207 -> [w222]
        tunnel: w206 -> [w221]
        tunnel: w205 -> [w219]
        tunnel: w204 -> [w217]
        shift-right: [w215] -> w203
        shift-left: w202 -> [w216]
        shift-right: [w213] -> w200
        shift-left: w201 -> [w214]
        shift-right: [w212] -> _
        shift-left: _ -> [w211]
        stop <- w224 stop-if-true
        n91 = stacked-sequence {
          seq-local: [w245 _ _] -> [_ w399 _]
          seq-local: [w253 _ _] -> [_ w398 _]
          seq-local: [w272 _ _] -> [_ w392 w945]
          seq-local: [w267 _ _] -> [_ w391 _]
          seq-local: [w243 _ _] -> [_ w381 w943]
          seq-local: [w241 _ _] -> [_ w382 _]
          seq-local: ["SavePath" _ _] -> [_ w378 _]
          tunnel: w225 -> [_ w401 _]
          tunnel: [_ w400 _] -> w224
          tunnel: w223 -> [w237 _ _]
          tunnel: w218 -> [_ w383 _]
          tunnel: w222 -> [_ w394 _]
          tunnel: w221 -> [_ w393 _]
          tunnel: "Software Gate" -> [w268 w390 _]
          tunnel: w219 -> [_ _ _]
          tunnel: w217 -> [w227 w389 _]
          tunnel: w216 -> [w257 _ _]
          tunnel: [_ w379 _] -> w215
          tunnel: w214 -> [w242 w380 _]
          tunnel: [w241 _ _] -> w213
          tunnel: [_ w377 _] -> w212
          tunnel: w211 -> [_ w376 _]
          frame #0 {
            # "Precalc for sector images"
            # "RF lines"
            # "Set up sampling rete and delay"
            # "These are microseconds"
            n92 = property on="Probe" class="Ring (strict)"() -> ("NumItems"=w261:u32, "Value"=w262:u16)  [unwired: 2 in, 2 out]
            n93 = global write "MotionGlobals.vi" "SavePath"("SavePath") -> ()
            n94 = Increment(x=w262) -> (x+1=w260:u16)
            n95 = call <vilib>:"Check if File or Folder Exists.vi"("path"="SavePath") -> ("file or folder exists?"=w231:bool, "dup path"=w230:path)  [unwired: 8 in, 1 out]
            n96 = Equal?(x=w261, y=w260) -> (x = y?=w240:bool)
            n97 = Or(x=w240, y="Overide Gain?") -> (x .or. y?=w238:bool)
            n98 = case shown="False" w238 {
              tunnel: [w288 w306] -> w236
              tunnel: [w294 w305] -> w271
              tunnel: [w295 "Scan Info"] -> w267
              tunnel: [w292 w303] -> w264
              tunnel: [w293 w302] -> w263
              tunnel: w227 -> [w296 _]
              tunnel: w242 -> [w291 w301]
              tunnel: [w289 w301] -> w241
              tunnel: [w287 _] -> w228
              tunnel: ["Probe" _] -> w226
              frame False {
                n99 = call "ReadOrSaveCases-UTEX.vi"("Location"=w296, "Save(T)\\Read(F)"=FALSE ("Save(T)\\Read(F)")) -> ("CaseArray"=w298:T33)  [unwired: 8 in, 1 out]
                n100 = Index Array(array=w298, index="Probe") -> (element=w297:T34)
                n101 = Unbundle(w297) -> ("Distance between\nscan lines (mm)"=w290:sgl, "Acquistion Parameters"=w288:T3, "Timeout (s)"=w292:dbl, "Sector?"=w293:bool, "Filter Prams"=w294:T1, "Scan Info"=w295:T2, "UT340 Controls"=w287:T5)  [unwired: 1 out]
                n102 = Bundle By Name(cluster=w291, "Distance between\nscan lines (um)"=w290) -> (w289:T8)
              }
              frame True {
                n103 = local read "Timeout (s)"() -> (w303:dbl)
                n104 = local read "Acq Params"() -> (w306:T3)
                n105 = local read "Filter Prams"() -> (w305:T1)
                n106 = local read "Sector?"() -> (w302:bool)
                n107 = local write "Overide Gain?"(FALSE ("Overide Gain?")) -> ()
              }
            }
            n108 = case shown="False" w231 {
              tunnel: w230 -> [w279 _]
              frame False {
                n109 = Create Folder(path (use dialog)=w279) -> ()  [unwired: 2 in, 3 out]
              }
              frame True {
              }
            }
            n110 = Unbundle By Name(w236) -> ("Sampling Rate"=w273:dbl, "Ref Delay (ms)"=w250:dbl, "rf points per line"=w256:i32, "rf lines"=w252:i32, "Dig Scale"=w255:dbl)
            n111 = local write "Timeout (s)"(w264) -> ()
            n112 = local write "Sector?"(w263) -> ()
            n113 = property on="Filter Prams" class="Clust (strict)"("Value"=w271) -> ()  [unwired: 2 in, 2 out]
            n114 = property on="Scan Info" class="Clust (strict)"("Value"=w267) -> ()  [unwired: 2 in, 2 out]
            n115 = local write "Acq Params"(w236) -> ()
            n116 = property on="Pulser" class="Enum (strict)"() -> ("Value"=w229:T4)  [unwired: 2 in, 2 out]
            n117 = case shown="\"UTEX\"" w229 {
              tunnel: w228 -> [_ w278]
              tunnel: w226 -> [_ w277]
              frame Default {
              }
              frame "UTEX" {
                w274 = FALSE ("PULSE")
                n118 = Bundle By Name(cluster=w278, "PULSE"=w274) -> (w275:T5)
                n119 = property on="Acquire Data" class="Bool (strict)"("Value"=w274) -> ()  [unwired: 2 in, 2 out]
                n120 = call "RiversideRelaySetChannel.vi"("Transducer"=w277) -> ()  [unwired: 4 in, 3 out]
                n121 = call "UTEX Send Values MultiTry.vi"("UT340 Controls"=w275) -> ("UT340 Controls Out"=w276:T5)  [unwired: 3 in, 1 out]
                n122 = property on="UT340 Controls" class="Clust (strict)"("Value"=w276) -> ()  [unwired: 2 in, 2 out]
              }
            }
            n123 = expression code="x*1"(w252) -> (w270:i32)
            n124 = Select(t=w270, s=w268, f=w252) -> (s? t:f=w269:i32)
            n125 = expression code="x*1E6"(w273) -> (w249:dbl)
            n126 = Bundle By Name(cluster=w257, "Samp Rate (Hz)"=w249, "Digitizer delay (us)"=w250, "rf points per line"=w256, "lines per plane"=w252, "Voltage Scale"=w255) -> (w235:T28)
            n127 = case shown="\"AlazarTech\"" w237 {
              tunnel: w256 -> [w318 w351 w355]
              tunnel: w269 -> [w317 w346 w364]
              tunnel: [_ _ w365] -> w272
              tunnel: "Bang Trig" -> [w312 w342 w371]
              tunnel: T20 {"Source"=1, "Coupling"=0, "Slope"=0, "Level"=1500.0} ("Trigger") -> [w311 w340 w370]
              tunnel: T19 {"Voltage Scale"=0.0, "Offset"=0.0, "Coupling"=2} ("V scale") -> [w310 w339 w367]
              tunnel: w235 -> [w309 w334 w354]
              tunnel: [w307 w333 w352] -> w234
              frame "Acqiris Digitizer" {
                n128 = Unbundle By Name(w309) -> ("Voltage Scale"=w308:dbl, "Digitizer ID Cluster.Acqiris/Alazar/SP ID"=w320:u32[])
                n129 = expression code="x*1000*0.5/2"(w308) -> (w314:dbl)
                n130 = Index Array(array=w320) -> (element=w319:u32)  [unwired: 1 in]
                n131 = Bundle By Name(cluster=T20 {"Source"=0, "Coupling"=0, "Slope"=0, "Level"=1500.0} ("Trigger"), "Level"=w314) -> (w313:T20)
                n132 = Select(t=w313, s=w312, f=w311) -> (s? t:f=w307:T20)
                n133 = Bundle By Name(cluster=w310, "Voltage Scale"=w308) -> (w316:T19)
                n134 = disable-structure shown="Disabled" {
                  disable-tunnel: w319 -> [w332 _]
                  disable-tunnel: w318 -> [w330 _]
                  disable-tunnel: w317 -> [w329 _]
                  disable-tunnel: w316 -> [w328 _]
                  disable-tunnel: w309 -> [w323 _]
                  disable-tunnel: w308 -> [w322 _]
                  disable-tunnel: w307 -> [w321 _]
                  frame Disabled {
                    n135 = call "conSamp.vi"("Digitizer Settings"=w323, "InstrumentID"=w332) -> ("DUP ID"=w331:u32)  [unwired: 2 in, 1 out]
                    n136 = call <instrlib>:"Configure Memory Settings.vi"("Number of Samples (1000)"=w330, "Number of Segments (1)"=w329, "Instrument ID"=w331) -> ("error out"=w325:errorcluster, "dup Instrument ID"=w327:u32)  [unwired: 1 in, 2 out]
                    n137 = call "conTrig.vi"("error in"=w325, "Voltage Scale"=w322, "Trigger"=w321, "InstrumentID"=w327) -> ("error out"=w324:errorcluster, "dup id"=w326:u32)  [unwired: 1 in]
                    n138 = call "conVert.vi"("InstrumentID"=w326, "V scale"=w328, "error in"=w324) -> ()  [unwired: 3 in, 2 out]
                  }
                  frame Enabled {
                  }
                }
              }
              frame "NI Digitizer", Default {
                w348 = TRUE
                n139 = Unbundle By Name(w334) -> ("Digitizer ID Cluster.NI Instr Handles"=w347:refnum<k15>[], "Voltage Scale"=w336:dbl)
                n140 = expression code="x*1000*0.95/2"(w336) -> (w343:dbl)
                n141 = Index Array(array=w347) -> (element=w344:refnum<k15>)  [unwired: 1 in]
                n142 = Bundle By Name(cluster=T21 {"Source"=0, "Coupling"=3, "Slope"=0, "Level (mV)"=1500.0} ("Trigger Settings"), "Level (mV)"=w343) -> (w341:T21)
                n143 = property class="niScope"(reference=w344, "Channel Enabled"=w348, "Min Number of Points"=w351, "Number of Records"=w346, "Enable Records > Memory"=w348) -> (reference out=w350:refnum<k15>, error out=w349:errorcluster)  [unwired: 1 in]
                n144 = Select(t=w341, s=w342, f=w340) -> (s? t:f=w333:T20)
                n145 = call "NI conSamp.vi"("error in"=w349, "Digitizer Settings"=w334, "InstrumentID"=w350) -> ("DUP ID"=w335:refnum<k15>)  [unwired: 1 in, 1 out]
                n146 = Bundle By Name(cluster=w339, "Voltage Scale"=w336) -> (w338:T19)
                n147 = call "NIconTrig.vi"("Trigger"=w333, "InstrumentID"=w335) -> ("dup id"=w337:refnum<k15>)  [unwired: 1 in, 2 out]
                n148 = call "NIconVert.vi"("InstrumentID"=w337, "V scale"=w338) -> ()  [unwired: 2 in, 4 out]
              }
              frame "AlazarTech" {
                w363 = u32 1 items=["A"=1, "B"=2, "A + B"=3, "C"=4, "A + C"=5, "A + B"=6, "D"=8, "A + D"=9, "B + D"=10, "C + D"=12, "A + B + C + D"=15] ("Channel")
                (unwired) 4 ("BuffCount")
                (unwired) TRUE ("Enable Trigger Enable")
                # "Will use software frame synch so Enable Trigger Enable T"
                # "Need to start Acq"
                # "Alazar does not provide voltage scale info when reading data."
                n149 = Unbundle By Name(w354) -> ("Digitizer ID Cluster.Acqiris/Alazar/SP ID"=w373:u32[], "Voltage Scale"=w366:dbl)
                n150 = expression code="x*1000*0.99/2"(w366) -> (w372:dbl)
                n151 = Bundle By Name(cluster=T21 {"Source"=0, "Coupling"=2, "Slope"=0, "Level (mV)"=1500.0} ("Trigger Settings"), "Level (mV)"=w372) -> (w368:T21)
                n152 = Index Array(array=w373) -> (element=w360:u32)  [unwired: 1 in]
                n153 = Select(t=w368, s=w371, f=w370) -> (s? t:f=w352:T20)
                n154 = Bundle(cluster=w367, "Voltage Scale"=w366) -> (w353:T19)  [unwired: 2 in]
                n155 = call "Alazar_ChannelConfig - ATS-SDK.vi"("V scale"=w353, "Channel"=w363, "Handle in"=w360) -> ("error out"=w356:errorcluster, "Handle_Out"=w359:u32)  [unwired: 2 in, 1 out]
                n156 = call "Alazar_conTrig - ATS-SDK.vi"("error in (no error)"=w356, "Trigger"=w352, "Voltage Scale"=w366, "Handle in"=w359) -> ("error out"=w357:errorcluster, "Handle_Out"=w358:u32)  [unwired: 1 in]
                n157 = call "AlazarAcqPrep - ATS-SDK.vi"("Handle"=w358, "Digitizer Settings"=w354, "Channel"=w363, "rf points per line"=w355, "error in (no error)"=w357, "rf lines per buffer"=w364) -> ("Handle Out"=w362:u32, "AlazarCluster"=w365:T35, "error out"=w361:errorcluster)  [unwired: 6 in, 1 out]
                n158 = call "AlazarStartCapture.vi"("Handle"=w362, "error in (no error)"=w361) -> ()  [unwired: 3 out]
              }
            }
            n159 = flat-sequence {
              tunnel: [w280] -> w244
              tunnel: w233 -> [w284]
              tunnel: [w285] -> w245
              tunnel: w244 -> [w283]
              tunnel: [w284] -> w243
              tunnel: w241 -> [w282]
              frame #0 {
                n160 = expression code="x/1000"("c (m/s)") -> (w280:dbl)
              }
              frame #1 {
                n161 = call "PlotScalingParams.vi"("Motion Settings In"=w282, "c mm/mics"=w283, "Digitizer Settings"=w284) -> ("Cluster"=w285:T36)  [unwired: 6 in, 2 out]
              }
            }
            n162 = Bundle By Name(cluster=w235, "Trigger Settings"=w234) -> (w233:T28)
            n163 = Unbundle By Name(w245) -> ("Y Scale Offset"=w246:dbl)
            n164 = Unbundle By Name(w243) -> ("rf points per line"=w248:i32, "lines per plane"=w247:i32)
            n165 = Divide(x=w248, y=2) -> (x/y=w251:dbl)
            n166 = call "PreCalcSecDisplayParams.vi"("delay mm"=w246, "pixels in y"=w251, "Background Value"=-100.0 ("element"), "Digitizer Settings"=w243, "pixels in x"=w247) -> ("Cluster out"=w253:T37)  [unwired: 6 in]
          }
          frame #1 {
            # "save eye if selected"
            # "Get data and feed to other loop"
            n167 = Unbundle By Name(w381) -> ("bits A/D"=w384:i8, "Samp Rate (Hz)"=w385:dbl)
            n168 = Unbundle By Name(w383) -> ("DataBufferQ"=w396:refnum<queue>, "Stop"=w395:refnum<notifier>)
            n169 = expression code="x*1E-6"(w385) -> (w402:dbl)
            n170 = while {
              tunnel: w399 -> [w433]
              tunnel: [w430] -> w403
              tunnel: w378 -> [w432]
              tunnel: w401 -> [w431]
              tunnel: w398 -> [w428]
              tunnel: w402 -> [w427]
              tunnel: [w426] -> w400
              shift-right: [w424] -> _
              shift-left: _ -> [w425]
              tunnel: w383 -> [w423]
              tunnel: w393 -> [w421]
              tunnel: w394 -> [w420]
              tunnel: w391 -> [w419]
              tunnel: w390 -> [w418]
              tunnel: w389 -> [w415]
              tunnel: w384 -> [w414]
              tunnel: w382 -> [w412]
              tunnel: w380 -> [w411]
              tunnel: w381 -> [w413]
              tunnel: [w410] -> w379
              shift-right: [w409] -> w377
              shift-left: w376 -> [w408]
              i -> [w434]
              stop <- w430 stop-if-true
              n171 = local read "append letter"() -> (w422:i8)
              n172 = event shown="[8] \"Patient Info\": Value Change" {
                selector: _ -> [_ _ _ _ _ _ _ _ _ _ _ _ _ _ _ _ _ _ _ _ _ _ _]
                dyn-events: _ -> [_ _ _ _ _ _ _ _ _ _ _ _ _ _ _ _ _ _ _ _ _ _ _]
                timeout: 40 -> [_ _ _ _ _ _ _ _ _ _ _ _ _ _ _ _ _ _ _ _ _ _ _]
                tunnel: w434 -> [w453 _ _ _ _ _ _ _ _ _ _ _ _ _ _ _ _ _ _ _ _ _ _]
                tunnel: w433 -> [_ w574 _ _ _ _ _ _ _ _ _ _ _ _ _ _ _ _ _ _ _ _ _]
                tunnel: [_ _ _ _ w657 TRUE TRUE _ _ _ _ _ _ _ _ _ _ _ _ _ _ _ _] -> w430
                tunnel: w432 -> [w435 _ _ _ _ _ _ _ w692 _ _ _ _ _ _ w755 _ _ _ w834 _ _ _]
                tunnel: w431 -> [w452 _ _ _ _ _ _ _ _ _ _ _ _ _ _ _ _ _ _ _ _ _ _]
                tunnel: w428 -> [w451 w568 _ _ _ _ _ _ _ _ _ _ _ _ _ _ w777 _ _ _ _ _ _]
                tunnel: w427 -> [w450 _ _ _ _ _ _ _ _ _ _ _ _ _ _ _ _ _ _ _ _ _ _]
                tunnel: [_ _ _ _ w657 _ _ _ _ _ _ _ _ _ _ _ _ _ _ _ _ _ _] -> w426
                tunnel: w425 -> [w444 _ _ _ _ _ _ _ _ _ _ _ _ _ _ _ _ _ _ _ _ _ _]
                tunnel: [w443 _ _ _ _ _ _ _ _ _ _ _ _ _ _ _ _ _ _ _ _ _ _] -> w424
                tunnel: w423 -> [w449 _ _ _ w655 w661 w675 w686 _ _ _ _ _ _ _ w771 _ _ w828 w843 _ _ _]
                tunnel: w422 -> [w442 _ _ _ _ _ _ _ _ _ _ _ _ _ w747 w763 _ _ _ w844 _ _ _]
                tunnel: w421 -> [_ _ _ _ _ _ _ _ _ _ _ _ _ _ _ _ w779 w822 _ _ _ _ _]
                tunnel: w420 -> [_ _ _ _ _ _ _ _ _ _ _ _ _ _ _ _ w778 _ _ _ _ _ _]
                tunnel: w419 -> [w448 _ _ _ _ _ _ _ _ _ _ _ _ _ _ w758 _ _ _ w838 _ _ _]
                tunnel: w418 -> [_ _ _ w645 _ _ _ _ _ _ _ _ _ _ _ _ _ _ _ _ _ _ _]
                tunnel: T22 {"DataBufferQ"=refnum, "LastNQ"=refnum, "LastNBMPQ"=refnum, "SaveRawN"=refnum, "StopN"=refnum} ("Qs and Notis") -> [_ _ _ _ _ _ _ _ _ _ _ _ _ _ _ w767 _ _ _ w841 _ _ _]
                tunnel: "Sector?" -> [w441 w573 _ _ _ _ _ _ _ _ _ _ _ _ _ _ w775 _ _ _ _ _ _]
                tunnel: w415 -> [w436 w565 w634 _ _ _ _ _ w689 _ _ _ _ _ _ w753 w773 _ _ w831 w862 _ _]
                tunnel: w414 -> [w440 _ _ _ _ _ _ _ _ _ _ _ _ _ _ w761 _ _ _ w837 _ _ _]
                tunnel: w413 -> [w438 w571 w632 w644 w653 w659 w678 w681 w693 w701 w705 w712 w717 w730 w745 w759 w774 w821 w825 w836 w860 w883 w914]
                tunnel: w412 -> [w439 _ _ _ _ _ _ _ _ _ _ _ _ _ _ w760 _ _ _ _ w861 _ _]
                tunnel: w411 -> [_ _ _ _ _ _ w679 _ _ _ _ _ _ _ _ _ _ _ _ _ _ _ _]
                tunnel: [w438 w571 w632 w644 w653 w659 w666 w681 w693 w701 w705 w712 w717 w730 w745 w759 w774 w821 w825 w836 w860 w883 w914] -> w410
                tunnel: [_ w570 _ _ _ _ _ _ _ _ _ _ _ _ _ _ _ _ _ _ _ _ _] -> _
                tunnel: [w437 w569 w635 w643 w652 w658 w673 w680 w691 w699 w704 w711 w716 w729 w744 w756 w772 w820 w824 w835 w859 w881 w906] -> w409
                tunnel: w408 -> [w437 w569 w635 w643 w652 w658 w673 w680 w690 w700 w704 w711 w716 w729 w744 w756 w772 w820 w824 w835 w859 w881 w906]
                event Timeout {
                  n173 = event-data() -> ()  [unwired: 1 in, 1 out]
                  n174 = Unbundle By Name(w449) -> ("DataBufferQ"=w447:refnum<queue>)
                  n175 = Dequeue Element(queue=w447) -> (element=w446:T16)  [unwired: 2 in, 3 out]
                  n176 = Unbundle(w446) -> (w445:bool)  [unwired: 4 out]
                  "No data\nEntering\nQueue" <- w445
                  n177 = case shown="False" w445 {
                    tunnel: w453 -> [w472 _]
                    tunnel: w452 -> [w471 _]
                    tunnel: w451 -> [w470 _]
                    tunnel: w450 -> [w469 _]
                    tunnel: w449 -> [w468 _]
                    tunnel: w448 -> [w467 _]
                    tunnel: w446 -> [w465 _]
                    tunnel: w444 -> [w464 w564]
                    tunnel: [w463 w564] -> w443
                    tunnel: w442 -> [w461 _]
                    tunnel: w441 -> [w460 _]
                    tunnel: w440 -> [w459 _]
                    tunnel: w439 -> [w458 _]
                    tunnel: w438 -> [w457 _]
                    tunnel: w437 -> [w456 _]
                    tunnel: w436 -> [w455 _]
                    tunnel: w435 -> [w454 _]
                    frame False {
                      n178 = stacked-sequence {
                        tunnel: w472 -> [w499 w542]
                        tunnel: w471 -> [w497 _]
                        tunnel: w470 -> [w494 _]
                        tunnel: w469 -> [w493 _]
                        tunnel: w468 -> [w487 w540]
                        tunnel: w467 -> [_ w535]
                        tunnel: "Save Raw" -> [_ w537]
                        tunnel: w465 -> [w490 w536]
                        tunnel: w464 -> [w479 _]
                        tunnel: [w477 _] -> w463
                        tunnel: "Pause" -> [w476 w534]
                        tunnel: w461 -> [_ w531]
                        tunnel: w460 -> [w475 _]
                        tunnel: w459 -> [w473 w529]
                        tunnel: w458 -> [_ w528]
                        tunnel: w457 -> [_ w527]
                        tunnel: w456 -> [_ w524]
                        tunnel: w455 -> [_ w523]
                        tunnel: w454 -> [_ w522]
                        frame #0 {
                          # "set scale after first image"
                          # "Get and display data"
                          n179 = Unbundle(w490) -> ("gain"=w486:dbl, "wfm"=w485:i16[][])  [unwired: 3 out]
                          n180 = Increment(x=w499) -> (x+1=→"Current Image":i32)
                          n181 = call "SubMean.vi"("Bit Depth"=w473, "Scan Data In"=w485, "Samp Rate (MHz)"=w493, "Filter Prams"="Filter Prams", "Type of Mean"="Type of Mean") -> ("Array"=w498:dbl[][])  [unwired: 1 in, 2 out]
                          n182 = Unbundle By Name(w487) -> ("LastNQ"=w489:refnum<queue>)
                          n183 = case shown="False" w475 {
                            tunnel: [w510 w519] -> w495
                            tunnel: w498 -> [w509 w520]
                            tunnel: w497 -> [w508 w521]
                            tunnel: w494 -> [_ w518]
                            frame False {
                              # "Linear array data"
                              n184 = for {
                                tunnel: [w513] -> w510 mode=indexing
                                tunnel: w509 -> [w512] mode=indexing
                                tunnel: w508 -> [w511]
                                n185 = for {
                                tunnel: [w517] -> w513 mode=indexing
                                tunnel: w512 -> [w516] mode=indexing
                                tunnel: w511 -> [w514]
                                n186 = Absolute Value(x=w516) -> (abs(x)=w515:dbl)
                                n187 = Index Array(array=w514, index=w515) -> (element=w517:sgl)
                                }
                              }
                            }
                            frame True {
                              # "Convert to sector"
                              n188 = call "AvisoSectorConvert.vi"("output cluster"=w518, "Log Lookup"=w521, "Raw In"=w520) -> ("Sector out"=w519:dbl[][])  [unwired: 8 in]
                            }
                          }
                          n189 = Bundle("gain"=w486, "wfm"=w485) -> (w484:cluster{"gain":dbl, "wfm":i16[][]})  [unwired: 1 in]
                          n190 = case shown="True" w476 {
                            tunnel: w489 -> [w502 w505]
                            tunnel: [w502 w504] -> w488
                            tunnel: w484 -> [_ w503]
                            frame False {
                            }
                            frame True {
                              n191 = Lossy Enqueue Element(queue=w505, element=w503) -> (queue out=w504:refnum<queue>)  [unwired: 1 in, 3 out]
                            }
                          }
                          n192 = Get Queue Status(queue=w488) -> (# elements in queue=w474:i32)  [unwired: 2 in, 7 out]
                          "In Queue" <- w474
                          n193 = case shown="2" w474 {
                            frame 0, Default {
                            }
                            frame 2 {
                              n194 = stacked-sequence {
                                frame #0 {
                                n195 = local read "distance?"() -> (w500:bool)
                                n196 = property on="distance?" class="Bool (strict)"("Val(Sgnl)"=w500) -> ()  [unwired: 2 in, 2 out]
                                }
                                frame #1 {
                                n197 = property on="1:1\nAspect" class="Bool (strict)"("Val(Sgnl)"=FALSE ("Value (Signaling)")) -> ()  [unwired: 2 in, 2 out]
                                }
                              }
                            }
                          }
                          n198 = flat-sequence {
                            tunnel: w495 -> [w506]
                            tunnel: [w507] -> w477
                            frame #0 {
                              "Raw data" <- w506
                            }
                            frame #1 {
                              n199 = Tick Count (ms)() -> (millisecond timer value=w507:u32)
                            }
                          }
                          n200 = Subtract(x=w477, y=w479) -> (x-y=w483:u32)
                          n201 = To Double Precision Float(number=w483) -> (double precision float=w482:dbl)
                          n202 = expression code="1000/x"(w482) -> (w481:dbl)
                          n203 = call <vilib>:"Mean PtByPt.vi"("x"=w481, "sample length"=10) -> ("mean"=→"fps":dbl)  [unwired: 2 in, 1 out]
                        }
                        frame #1 {
                          w530 = "_" ("string")
                          # "Save jpg if selected"
                          n204 = Type Cast(x=w531) -> (*(type *) &x=w533:string)  [unwired: 1 in]
                          n205 = call "PathCreate.vi"("Location"=w523, "Patient Info"=w524, "base path"=w522) -> ("FileName"=w525:string, "appended path"=w526:path)  [unwired: 7 in]
                          n206 = invoke on="Raw data" class="IntGraph (strict)" method="Get Image"("image depth"=24) -> ("image data"=w538:T18)  [unwired: 5 in, 5 out]
                          n207 = Concatenate Strings(w525, w530, w533, w530) -> (w532:string)
                          n208 = case shown="True" w537 {
                            tunnel: w542 -> [_ w547]
                            tunnel: w532 -> [_ w556]
                            tunnel: w538 -> [_ w558]
                            tunnel: w536 -> [_ w557]
                            tunnel: w535 -> [_ w553]
                            tunnel: w529 -> [_ w552]
                            tunnel: w528 -> [_ w551]
                            tunnel: w527 -> [_ w550]
                            tunnel: w526 -> [_ w545]
                            tunnel: w524 -> [_ w546]
                            frame False {
                            }
                            frame True {
                              n209 = Unbundle(w557) -> ("gain"=w555:dbl, "wfm"=w554:i16[][])  [unwired: 3 out]
                              n210 = property on="Name add on" class="Ring (strict)"() -> ("RingText.Text"=w548:string)  [unwired: 2 in, 2 out]
                              n211 = case shown="True" FALSE {
                                tunnel: w558 -> [_ w563]
                                tunnel: w556 -> [_ w562]
                                tunnel: w547 -> [_ w561]
                                tunnel: w548 -> [_ w560]
                                tunnel: w545 -> [_ w559]
                                frame False {
                                }
                                frame True {
                                n212 = call "RT_Save_JPG.vi"("base path"=w559, "Append Extra"=w560, "Movie Name"=w562, "Frame"=w561, "image data"=w563) -> ()  [unwired: 7 in]
                                }
                              }
                              n213 = call "RT_Save_EYE.vi"("Data"=w554, "Eye Name"=w556, "Save Directory"=w545, "Digitizer Gain"=w555, "Patient Info"=w546, "Frame"=w547, "Scan Info"=w553, "Digitizer Settings"=w550, "bits A/D"=w552, "File Append"=w548, "Motion Settings"=w551) -> ()  [unwired: 5 in]
                            }
                          }
                          n214 = Unbundle By Name(w540) -> ("LastN_JPG_Q"=w539:refnum<queue>)
                          n215 = case shown="True" w534 {
                            tunnel: w539 -> [_ w544]
                            tunnel: w538 -> [_ w543]
                            frame False {
                            }
                            frame True {
                              n216 = Lossy Enqueue Element(queue=w544, element=w543) -> ()  [unwired: 1 in, 4 out]
                            }
                          }
                        }
                      }
                    }
                    frame True {
                      # "If time out or error in acquisition don't do anything"
                    }
                  }
                }
                event "distance?", "Sector?": Value Change {
                  w572 = u8 1 ("X Scale.Scale Fit")
                  # "Choose distance or index scales"
                  n217 = event-data() -> ()  [unwired: 1 in, 3 out]
                  n218 = property on="Probe" class="Ring (strict)"() -> ("Value"=w566:u16)  [unwired: 2 in, 2 out]
                  n219 = case shown="\"HSS\"" w565 {
                    tunnel: [T23 [{"Active Cursor"=0, "Cursor.Cursor Color"=16711680, "Cursor.Cursor Position:Cursor Y"=2.0, "Cursor.Cursor Position:Cursor X"=0.0, "Cursor.Cursor Style"=6, "Cursor.Line Style"=0, "Cursor.Line Width"=2, "Cursor.Visible"=TRUE}, {"Active Cursor"=1, "Cursor.Cursor Color"=16860, "Cursor.Cursor Position:Cursor Y"=2.2, "Cursor.Cursor Position:Cursor X"=0.0, "Cursor.Cursor Style"=6, "Cursor.Line Style"=0, "Cursor.Line Width"=2, "Cursor.Visible"=TRUE}] w582] -> w567
                    tunnel: w566 -> [_ w581]
                    frame Default {
                    }
                    frame "HSS" {
                      n220 = case shown="1" w581 {
                        tunnel: [T23 [{"Active Cursor"=0, "Cursor.Cursor Color"=6618880, "Cursor.Cursor Position:Cursor Y"=1.3, "Cursor.Cursor Position:Cursor X"=0.0, "Cursor.Cursor Style"=6, "Cursor.Line Style"=0, "Cursor.Line Width"=2, "Cursor.Visible"=TRUE}, {"Active Cursor"=1, "Cursor.Cursor Color"=16860, "Cursor.Cursor Position:Cursor Y"=2.35, "Cursor.Cursor Position:Cursor X"=0.0, "Cursor.Cursor Style"=6, "Cursor.Line Style"=0, "Cursor.Line Width"=2, "Cursor.Visible"=TRUE}] T23 [{"Active Cursor"=0, "Cursor.Cursor Color"=6618880, "Cursor.Cursor Position:Cursor Y"=11.5, "Cursor.Cursor Position:Cursor X"=0.0, "Cursor.Cursor Style"=6, "Cursor.Line Style"=0, "Cursor.Line Width"=2, "Cursor.Visible"=TRUE}, {"Active Cursor"=1, "Cursor.Cursor Color"=16860, "Cursor.Cursor Position:Cursor Y"=12.7, "Cursor.Cursor Position:Cursor X"=0.0, "Cursor.Cursor Style"=6, "Cursor.Line Style"=0, "Cursor.Line Width"=2, "Cursor.Visible"=TRUE}]] -> w582
                        frame 1 {
                        }
                        frame 0, Default {
                        }
                      }
                    }
                  }
                  n221 = case shown="True" "distance?" {
                    tunnel: [w595 w604] -> w579
                    tunnel: [w594 w603] -> w578
                    tunnel: [w595 w602] -> w577
                    tunnel: [w594 w601] -> w576
                    tunnel: w574 -> [_ w599]
                    tunnel: w573 -> [_ w597]
                    tunnel: w568 -> [_ w598]
                    tunnel: w565 -> [_ w596]
                    frame False {
                      w594 = 1
                      w595 = 0
                    }
                    frame True {
                      n222 = Unbundle(w599) -> ("Y Scale Offset"=w608:dbl, "Y Scale Multi"=w607:dbl, "X Scale Offset"=w606:dbl, "X Scale Multi"=w605:dbl, "Gate Distance"=w600:dbl)
                      n223 = case shown="True" w597 {
                        tunnel: w608 -> [w613 w631]
                        tunnel: w607 -> [w611 _]
                        tunnel: w606 -> [w615 _]
                        tunnel: w605 -> [w617 _]
                        tunnel: [w614 0.0 ("X Scale.Offset and Multiplier:Offset")] -> w604
                        tunnel: [w616 w627] -> w603
                        tunnel: [w612 w631] -> w602
                        tunnel: [w610 w626] -> w601
                        tunnel: w600 -> [_ _]
                        tunnel: w598 -> [_ w628]
                        tunnel: w596 -> [w609 _]
                        frame False {
                          n224 = case shown="\"Aline\"" w609 {
                            tunnel: w617 -> [w621 _]
                            tunnel: [w621 1.0 ("t")] -> w616
                            tunnel: w615 -> [w620 _]
                            tunnel: [w620 0.0 ("X Scale Offset")] -> w614
                            tunnel: w613 -> [w619 w623]
                            tunnel: [w619 w623] -> w612
                            tunnel: [w618 w622] -> w610
                            tunnel: w611 -> [w618 w622]
                            frame "CUMC", Default {
                            }
                            frame "Aline" {
                            }
                          }
                        }
                        frame True {
                          # "sector"
                          n225 = Unbundle(w628) -> ("scales"=w629:cluster{"inc x (mm)":dbl, "inc y (mm)":dbl})  [unwired: 6 out]
                          n226 = Unbundle(w629) -> ("inc x (mm)"=w627:dbl, "inc y (mm)"=w626:dbl)
                        }
                      }
                    }
                  }
                  n227 = for {
                    tunnel: w567 -> [w593] mode=indexing
                    n228 = Unbundle By Name(w593) -> ("Active Cursor"=w592:u32, "Cursor.Cursor Color"=w591:u32, "Cursor.Cursor Position:Cursor Y"=w590:dbl, "Cursor.Cursor Position:Cursor X"=w589:dbl, "Cursor.Cursor Style"=w588:u8, "Cursor.Line Style"=w587:u8, "Cursor.Line Width"=w586:u8, "Cursor.Visible"=w585:bool)
                    n229 = property on="Raw data" class="IntGraph (strict)"("Active Cursor"=w592, "Cursor.Cursor Color"=w591, "Cursor.Cursor Y"=w590, "Cursor.Cursor X"=w589, "Cursor.Cursor Style"=w588, "Cursor.LineStyle"=w587, "Cursor.LineWidth"=w586, "Cursor.Visible"=w585) -> ()  [unwired: 2 in, 2 out]
                  }
                  n230 = property on="Raw data" class="IntGraph (strict)"("X Scale.Offset and Multiplier:Offset"=w579, "X Scale.Offset and Multiplier:Multiplier"=w578, "Y Scale.Offset and Multiplier:Offset"=w577, "Y Scale.Offset and Multiplier:Multiplier"=w576, "XScale.ScaleFit"=w572, "YScale.ScaleFit"=w572) -> (error out=w570:errorcluster)  [unwired: 2 in, 1 out]
                }
                event "Acquire Data": Value Change {
                  # "F12 is current turn on key. Board spins and times out unti pressed"
                  n231 = event-data() -> ("NewVal"=w633:bool)  [unwired: 1 in]
                  n232 = case shown="\"HSS\"" w634 {
                    tunnel: w633 -> [w638 w642]
                    tunnel: w632 -> [w637 _]
                    frame "Aline", Default {
                      n233 = Unbundle By Name(w637) -> ("Digitizer ID Cluster.Acqiris/Alazar/SP ID"=w639:u32[])
                      n234 = Boolean To (0,1)(Boolean=w638) -> (0, 1=w641:i16)
                      n235 = Index Array(array=w639) -> (element=w640:u32)  [unwired: 1 in]
                      n236 = call "AlazarConfigureAuxIO.vi"("Parameter"=w641, "Mode"=u32 14, "Handle"=w640) -> ()  [unwired: 1 in, 3 out]
                    }
                    frame "HSS" {
                      n237 = property on="Acquire Data" class="Bool (strict)"("Value"=w642) -> ()  [unwired: 2 in, 2 out]
                      n238 = property on="PULSE" class="Bool (strict)"("Val(Sgnl)"=w642) -> ()  [unwired: 2 in, 2 out]
                    }
                  }
                }
                event "LowTime", "Gate Length": Value Change {
                  n239 = event-data() -> ()  [unwired: 1 in, 1 out]
                  n240 = case shown="False" w645 {
                    frame False {
                      n241 = flat-sequence {
                        tunnel: refnum<k21> "QuantGate" ("task in") -> [w649]
                        tunnel: [w648] -> w647
                        tunnel: w647 -> [_]
                        frame #0 {
                          n242 = call <vilib>:"DAQmx Stop Task.vi"("task/channels in"=w649) -> ("task out"=w648:refnum<k21>)  [unwired: 13 in, 1 out]
                        }
                        frame #1 {
                          n243 = call "FrameSync.vi"("LowTime"="LowTime", "Gate Length"="Gate Length") -> ()  [unwired: 8 in, 2 out]
                        }
                      }
                    }
                    frame True {
                    }
                  }
                }
                event "stop": Value Change {
                  w657 = TRUE
                  n244 = event-data() -> ()  [unwired: 1 in, 2 out]
                  n245 = Unbundle By Name(w655) -> ("Stop"=w654:refnum<notifier>)
                  n246 = Send Notification(notification=TRUE, notifier=w654) -> ()  [unwired: 1 in, 2 out]
                }
                event "Probe", "Bang Trig", "Software Gate", "c (m/s)", "Acq Params", "SavePath": Value Change {
                  # "restart loops if new probe selected"
                  # "Restart loops with new digitizer settings"
                  n247 = event-data() -> ()  [unwired: 1 in, 1 out]
                  n248 = Unbundle By Name(w661) -> ("Stop"=w660:refnum<notifier>)
                  n249 = Send Notification(notification=TRUE, notifier=w660) -> ()  [unwired: 1 in, 2 out]
                }
                event "SetDig": Value Change {
                  n250 = event-data() -> ()  [unwired: 1 in, 1 out]
                  n251 = Unbundle By Name(w675) -> ("Stop"=w676:refnum<notifier>)
                  n252 = Send Notification(notification=TRUE, notifier=w676) -> ()  [unwired: 1 in, 2 out]
                  n253 = call "SetUpDigi.vi"("Digitizer Settings"=w678, "Motion Settings In"=w679, "QAM Gate?"=TRUE) -> ("Digitizer Settings Out"=w666:T28, "RF data Sampling Out"=w667:T38)  [unwired: 10 in, 5 out]
                  n254 = Unbundle By Name(w667) -> ("Sampling Rate"=w668:dbl, "Ref Delay (ms)"=w672:dbl, "rf points per line"=w671:i32)
                  n255 = Unbundle By Name(w666) -> ("lines per plane"=w670:i32, "Voltage Scale"=w669:dbl)
                  n256 = expression code="x*1E6"(w668) -> ()  [unwired: 1 out]
                  n257 = Bundle("Sampling Rate"=w668, "Ref Delay (ms)"=w672, "rf points per line"=w671, "lines per plane"=w670, "Voltage Scale"=w669) -> (w665:T39)  [unwired: 1 in]
                  n258 = local write "Acq Params"(w665) -> ()
                }
                event "Gain": Value Change {
                  # "Restart loops with new gain setting"
                  # "Use this to force selected gain."
                  n259 = event-data() -> ()  [unwired: 1 in, 6 out]
                  n260 = property on="Acq Params" class="Clust (strict)"() -> ("Value"=w683:T3)  [unwired: 2 in, 2 out]
                  n261 = Unbundle By Name(w686) -> ("Stop"=w685:refnum<notifier>)
                  n262 = Bundle By Name(cluster=w683, "Dig Scale"="Gain") -> (w682:T3)
                  n263 = Send Notification(notification=TRUE, notifier=w685) -> ()  [unwired: 1 in, 2 out]
                  n264 = property on="Acq Params" class="Clust (strict)"("Value"=w682) -> ()  [unwired: 2 in, 2 out]
                  n265 = local write "Overide Gain?"(TRUE ("Overide Gain?")) -> ()
                }
                event "Patient Info": Value Change {
                  n266 = event-data() -> ()  [unwired: 1 in, 2 out]
                  n267 = call "Info.vi"("Location"=w689, "base path"=w692, "Patient Info In"=w690) -> ("NewCase?"=w694:bool, "FileName"=→"File Name":string, "Patient Info Out"=w691:T40)  [unwired: 6 in]
                  n268 = property on="Patient Info" class="Bool (strict)"("Value"=FALSE ("Patient Info")) -> ()  [unwired: 2 in, 2 out]
                  n269 = Unbundle By Name(w691) -> ("Plane"=w697:i8)
                  n270 = case shown="True" w694 {
                    frame False {
                    }
                    frame True {
                      # "Rest Letter Index"
                      n271 = local write "append letter"(i8 65 ("append letter")) -> ()
                    }
                  }
                  n272 = local write "Plane"(w697) -> ()
                }
                event "Plane": Mouse Up; "Scan Location": Value Change {
                  n273 = event-data() -> ()  [unwired: 1 in, 1 out]
                  n274 = Bundle By Name(cluster=w700, "Plane"="Plane", "Scan Location"="Scan Location") -> (w699:T40)
                }
                event "dB Range": Value Change {
                  n275 = event-data() -> ("NewVal"=w706:cluster{i32, i32})  [unwired: 1 in, 1 out]
                  n276 = Unbundle(w706) -> (w708:i32, w709:i32)
                  n277 = property on="Raw data" class="IntGraph (strict)"() -> ("ZScale.Range"=w707:T41)  [unwired: 2 in, 2 out]
                  n278 = Bundle By Name(cluster=w707, "Minimum"=w709, "Maximum"=w708) -> (w710:T41)
                  n279 = property on="Raw data" class="IntGraph (strict)"("ZScale.Range"=w710) -> ()  [unwired: 2 in, 2 out]
                }
                event "Visible": Value Change {
                  n280 = event-data() -> ("NewVal"=w713:bool)  [unwired: 1 in, 1 out]
                  n281 = property on="Raw data" class="IntGraph (strict)"("Active Cursor"=u32 0, "Cursor.Visible"=w713, "Active Cursor"=u32 1, "Cursor.Visible"=w713) -> ()  [unwired: 2 in, 2 out]
                }
                event "Center": Value Change {
                  n282 = event-data() -> ()  [unwired: 1 in, 2 out]
                  n283 = property on="Raw data" class="IntGraph (strict)"() -> ("XScale.Maximum"=w718:dbl, "XScale.Minimum"=w719:dbl, "YScale.Maximum"=w720:dbl, "YScale.Minimum"=w721:dbl)  [unwired: 2 in, 2 out]
                  n284 = Add(x=w718, y=w719) -> (x+y=w722:dbl)
                  n285 = Add(x=w720, y=w721) -> (x+y=w723:dbl)
                  n286 = expression code="x/2"(w722) -> (w724:dbl)
                  n287 = expression code="x/2"(w723) -> (w725:dbl)
                  n288 = Bundle(w724, w725) -> (w728:cluster{dbl, dbl})  [unwired: 1 in]
                  n289 = property on="Raw data" class="IntGraph (strict)"("Active Cursor"=u32 0, "Cursor.Cursor Position"=w728, "Active Cursor"=u32 1, "Cursor.Cursor Position"=w728) -> ()  [unwired: 2 in, 2 out]
                }
                event "Raw data": Cursor Move {
                  n290 = event-data() -> ()  [unwired: 1 in, 1 out]
                  n291 = property on="Raw data" class="IntGraph (strict)"("Active Cursor"=u32 0, "Active Cursor"=u32 1) -> ("Cursor.Cursor Position"=w740:T42, "Cursor.Cursor Position"=w735:T42)  [unwired: 2 in, 2 out]
                  n292 = Subtract(x=w740, y=w735) -> (x-y=w736:T42)
                  n293 = Unbundle(w736) -> ("Cursor X"=w737:dbl, "Cursor Y"=w731:dbl)
                  n294 = Re/Im To Polar(2:w731, 3:w737) -> (1:w732:dbl)  [unwired: 1 out]
                  n295 = Number To Fractional String(number=w732, precision (6)=i16 2) -> (F-format string=w741:string)  [unwired: 2 in]
                  n296 = Concatenate Strings(w741, " mm") -> (w743:string)
                  n297 = property on="Raw data" class="IntGraph (strict)"("Active Cursor"=u32 0, "Cursor.Cursor Name"=w743) -> ()  [unwired: 2 in, 2 out]
                }
                event "Save Raw": Value Change {
                  n298 = event-data() -> ("NewVal"=w746:bool)  [unwired: 1 in]
                  n299 = case shown="False" w746 {
                    tunnel: w747 -> [w748 _]
                    frame False {
                      n300 = Increment(x=w748) -> (x+1=w749:i8)
                      n301 = local write "append letter"(w749) -> ()
                    }
                    frame True {
                    }
                  }
                }
                event "Save All Queue": Value Change {
                  w770 = i16 1
                  # "Save last N files in queue"
                  n302 = event-data() -> ()  [unwired: 1 in, 2 out]
                  n303 = Unbundle By Name(w771) -> ("LastNQ"=w766:refnum<queue>, "LastN_JPG_Q"=w765:refnum<queue>)
                  n304 = Bundle(cluster=w767, "LastNQ"=w766, "LastNBMPQ"=w765) -> (w764:T22)  [unwired: 3 in]
                  n305 = call "ReadOrSaveCases-UTEX.vi"("Location"=w753, "Save(T)\\Read(F)"=FALSE ("Save(T)\\Read(F)")) -> ("Case List"=w752:string[])  [unwired: 8 in, 1 out]
                  n306 = property on="Probe" class="Ring (strict)"() -> ("Value"=w750:u16)  [unwired: 2 in, 2 out]
                  n307 = property on="Name add on" class="Ring (strict)"() -> ("RingText.Text"=w757:string)  [unwired: 2 in, 2 out]
                  n308 = Bundle(w770, w770, "N to save"="N to save") -> (w768:cluster{i16, i16, "N to save":u16})  [unwired: 1 in]
                  n309 = Index Array(array=w752, index=w750) -> (element=w751:string)
                  n310 = call "SaveQueueN.vi"("Slider Indexes"=w768, "Qs and Notis"=w764, "Location"=w753, "Append Extra"=w757, "append letter"=w763, "bits A/D"=w761, "Probe Name"=w751, "Patient Info"=w756, "Scan Info"=w758, "base path"=w755, "Motion Settings"=w760, "Digitizer Settings"=w759) -> ("append letter out"=w762:i8)  [unwired: 7 in]
                  n311 = local write "append letter"(w762) -> ()
                }
                event "1:1\nAspect": Value Change {
                  n312 = event-data() -> ()  [unwired: 1 in, 2 out]
                  n313 = case shown="\"SERI\", Default" w773 {
                    tunnel: w779 -> [_ w788]
                    tunnel: w778 -> [_ w787]
                    tunnel: w777 -> [_ w784]
                    tunnel: w775 -> [_ w783]
                    tunnel: w774 -> [_ w780]
                    frame "Aline", "HSS" {
                    }
                    frame "SERI", Default {
                      w782 = u8 1 ("X Scale.Scale Fit")
                      n314 = case shown="True" w783 {
                        tunnel: [w800 w803] -> w786
                        tunnel: [w801 w804] -> w785
                        tunnel: w784 -> [_ w805]
                        tunnel: w780 -> [w802 _]
                        frame False {
                          n315 = Unbundle By Name(w802) -> ("lines per plane"=w801:i32, "rf points per line"=w800:i32)
                        }
                        frame True {
                          n316 = Unbundle(w805) -> ("pixels in x"=w804:i16, "pixels in y"=w803:i16)  [unwired: 5 out]
                        }
                      }
                      n317 = property on="Raw data" class="IntGraph (strict)"() -> ("X Scale.Offset and Multiplier:Multiplier"=w789:dbl, "Y Scale.Offset and Multiplier:Multiplier"=w790:dbl)  [unwired: 2 in, 2 out]
                      n318 = Unbundle(w787) -> ("Width"=w797:u32, "Height"=w799:u32)
                      n319 = Multiply(x=w785, y=w789) -> (x*y=w791:dbl)
                      n320 = Multiply(x=w790, y=w786) -> (x*y=w792:dbl)
                      n321 = Divide(x=w797, y=w791) -> (x/y=w793:dbl)
                      n322 = Divide(x=w799, y=w792) -> (x/y=w794:dbl)
                      n323 = Divide(x=w793, y=w794) -> (x/y=w798:dbl)
                      n324 = Greater?(x=w798, y=1.0) -> (0:w795:bool)
                      n325 = case shown="True" w795 {
                        tunnel: w797 -> [_ w819]
                        tunnel: w798 -> [w812 w818]
                        tunnel: w799 -> [w811 _]
                        tunnel: w788 -> [w806 w817]
                        tunnel: [w807 w813] -> w781
                        frame False {
                          n326 = Multiply(x=w811, y=w812) -> (x*y=w808:dbl)
                          n327 = Unbundle By Name(w806) -> ("Top"=w810:i16)
                          n328 = Add(x=w810, y=w808) -> (x+y=w809:dbl)
                          n329 = Bundle By Name(cluster=w806, "Bottom"=w809) -> (w807:T13)
                        }
                        frame True {
                          n330 = Unbundle By Name(w817) -> ("Left"=w815:i16)
                          n331 = Divide(x=w819, y=w818) -> (x/y=w816:dbl)
                          n332 = Add(x=w815, y=w816) -> (x+y=w814:dbl)
                          n333 = Bundle By Name(cluster=w817, "Right"=w814) -> (w813:T13)
                        }
                      }
                      n334 = property on="Raw data" class="IntGraph (strict)"("Plot Bounds"=w781, "XScale.ScaleFit"=w782, "YScale.ScaleFit"=w782) -> ()  [unwired: 2 in, 2 out]
                    }
                  }
                  n335 = local write "1:1\nAspect"(FALSE ("1:1\nAspect")) -> ()
                }
                event "Fill\nSpace": Value Change {
                  w823 = u8 1 ("X Scale.Scale Fit")
                  n336 = event-data() -> ()  [unwired: 1 in, 6 out]
                  n337 = property on="Raw data" class="IntGraph (strict)"("Plot Bounds"=w822, "XScale.ScaleFit"=w823, "YScale.ScaleFit"=w823) -> ()  [unwired: 2 in, 2 out]
                }
                event "Flush Queue": Value Change {
                  n338 = event-data() -> ()  [unwired: 1 in, 6 out]
                  n339 = Unbundle By Name(w828) -> ("LastNQ"=w827:refnum<queue>, "LastN_JPG_Q"=w826:refnum<queue>)
                  n340 = Flush Queue(queue=w826) -> ()  [unwired: 1 in, 3 out]
                  n341 = Flush Queue(queue=w827) -> ()  [unwired: 1 in, 3 out]
                }
                event "View Queue": Value Change {
                  # "Save files baed on queue selection"
                  n342 = event-data() -> ()  [unwired: 1 in, 6 out]
                  n343 = Unbundle By Name(w843) -> ("LastNQ"=w840:refnum<queue>, "LastN_JPG_Q"=w839:refnum<queue>)
                  n344 = Bundle(cluster=w841, "LastNQ"=w840, "LastNBMPQ"=w839) -> (w842:T22)  [unwired: 3 in]
                  n345 = call "ReadOrSaveCases-UTEX.vi"("Location"=w831, "Save(T)\\Read(F)"=FALSE ("Save(T)\\Read(F)")) -> ("Case List"=w832:string[])  [unwired: 8 in, 1 out]
                  n346 = property on="Probe" class="Ring (strict)"() -> ("Value"=w830:u16)  [unwired: 2 in, 2 out]
                  n347 = call "ViewQueue.vi"("Image queue"=w839) -> ("Slider Indexes"=w846:cluster{i16, i16, i16}, "Save?"=w845:bool)  [unwired: 3 in]
                  n348 = Index Array(array=w832, index=w830) -> (element=w829:string)
                  n349 = case shown="True" w845 {
                    tunnel: w844 -> [_ w858]
                    tunnel: w846 -> [_ w857]
                    tunnel: w842 -> [_ w856]
                    tunnel: w837 -> [_ w855]
                    tunnel: w838 -> [_ w854]
                    tunnel: w836 -> [_ w852]
                    tunnel: w835 -> [_ w850]
                    tunnel: w834 -> [_ w849]
                    tunnel: w831 -> [_ w848]
                    tunnel: w829 -> [_ w847]
                    frame False {
                    }
                    frame True {
                      n350 = property on="Name add on" class="Ring (strict)"() -> ("RingText.Text"=w851:string)  [unwired: 2 in, 2 out]
                      n351 = call "SaveQueueN.vi"("Slider Indexes"=w857, "Qs and Notis"=w856, "Location"=w848, "Append Extra"=w851, "append letter"=w858, "bits A/D"=w855, "Probe Name"=w847, "Patient Info"=w850, "Scan Info"=w854, "base path"=w849, "Digitizer Settings"=w852) -> ("append letter out"=w853:i8)  [unwired: 8 in]
                      n352 = local write "append letter"(w853) -> ()
                    }
                  }
                }
                event "Save Setting Profile": Value Change {
                  # "Add profile case but check that Custom settings is selected."
                  n353 = event-data() -> ()  [unwired: 1 in, 1 out]
                  n354 = property on="Probe" class="Ring (strict)"() -> ("Value"=w866:u16, "NumItems"=w864:u32)  [unwired: 2 in, 2 out]
                  n355 = Increment(x=w866) -> (x+1=w863:u16)
                  n356 = Equal?(x=w863, y=w864) -> (x = y?=w865:bool)
                  n357 = case shown="True" w865 {
                    tunnel: w863 -> [_ w872]
                    tunnel: w862 -> [_ w871]
                    tunnel: w861 -> [_ w870]
                    frame False {
                    }
                    frame True {
                      n358 = local read "Acq Params"() -> (w868:T3)
                      n359 = Unbundle By Name(w870) -> ("Distance between\nscan lines (um)"=w869:sgl)
                      n360 = local read "Filter Prams"() -> (w876:T1)
                      n361 = local read "Timeout (s)"() -> (w878:dbl)
                      n362 = local read "Scan Info"() -> (w875:T2)
                      n363 = local read "Sector?"() -> (w877:bool)
                      n364 = property on="UT340 Controls" class="Clust (strict)"() -> ("Value"=w867:T5)  [unwired: 2 in, 2 out]
                      n365 = call "Prompt User for Input"() -> ("New Case Name"=w874:string)  [unwired: 17 in, 2 out]
                      n366 = Bundle("New Case Name"=w874, "Distance between\nscan lines (um)"=w869, "Acq Params"=w868, "Timeout (s)"=w878, "Sector?"=w877, "Filter Prams"=w876, "Scan Info"=w875, "Value"=w867) -> (w873:T43)  [unwired: 1 in]
                      n367 = call "ReadOrSaveCases-UTEX.vi"("Location"=w871, "New Case"=w873, "Save(T)\\Read(F)"=TRUE ("Save(T)\\Read(F)")) -> ("Case List"=w879:string[])  [unwired: 7 in, 1 out]
                      n368 = property on="Probe" class="Ring (strict)"("Strings []"=w879, "Value"=w872) -> ()  [unwired: 2 in, 2 out]
                    }
                  }
                }
                event Value Change {
                  n369 = event-data() -> ()  [unwired: 1 in, 6 out]
                  n370 = case shown="\"UTEX\"" "Pulser" {
                    frame Default {
                    }
                    frame "UTEX" {
                      n371 = node-c288(i64 75 ("Period")) -> (w888:T24)
                      n372 = timed-loop {
                        timing: w888 -> [_]
                        timing-out: [_] -> w887
                        tunnel: ["UT340 Controls"] -> w885
                        i -> [w896]
                        stop <- w894 continue-if-true
                        n373 = node-c288() -> ()  [unwired: 1 in, 1 out]
                        n374 = global read "PulserGlobals.vi" "UTEX VISA"() -> (w892:refnum<visa-resource-name>)
                        n375 = call "ReadCurrentSettings.vi"("VISA Refnum in"=w892) -> ("error out"=w890:errorcluster, "UT340 Controls"=w891:T5)  [unwired: 8 in, 1 out]
                        n376 = Not Equal?(x="UT340 Controls", y=w891) -> (x != y?=w899:T44)
                        n377 = call "UTEX Send.vi"("error in"=w890, "Changed Values?"=w899, "UT340 Controls"="UT340 Controls") -> ()  [unwired: 8 in, 1 out]
                        n378 = Cluster To Array(cluster=w899) -> (array=w897:bool[])
                        n379 = Or Array Elements(Boolean array=w897) -> (logical OR=w898:bool)
                        n380 = Greater?(x=w896, y=10) -> (0:w893:bool)
                        n381 = node-c288() -> ()  [unwired: 1 out]
                        n382 = And(x=w893, y=w898) -> (x .and. y?=w894:bool)
                      }
                      n383 = Unbundle By Name(w885) -> ("PULSE"=w884:bool)
                      n384 = node-c288(w887) -> ()
                      n385 = property on="Acquire Data" class="Bool (strict)"("Value"=w884) -> ()  [unwired: 2 in, 2 out]
                    }
                  }
                }
                event Key Down {
                  n386 = event-data() -> ("Char"=w909:i16, "VKey"=w913:T27)  [unwired: 1 in]
                  n387 = Equal?(x=i16 32 ("y"), y=w909) -> (x = y?=w911:bool)
                  n388 = Equal?(x=w913, y=eventvkey."F12") -> (x = y?=w910:bool)
                  n389 = Or(x=w911, y=w910) -> (x .or. y?=w907:bool)
                  n390 = case shown="True" w907 {
                    frame False {
                    }
                    frame True {
                      n391 = property on="Pulser" class="Enum (strict)"() -> ("Value"=w915:T4)  [unwired: 2 in, 2 out]
                      n392 = case shown="Default" w915 {
                        frame Default {
                          n393 = property on="Acquire Data" class="Bool (strict)"() -> ("Value"=w917:bool)  [unwired: 2 in, 2 out]
                          n394 = Not(x=w917) -> (.not. x?=w916:bool)
                          n395 = property on="Acquire Data" class="Bool (strict)"("Val(Sgnl)"=w916) -> ()  [unwired: 2 in, 2 out]
                        }
                        frame "UTEX" {
                          n396 = property on="PULSE" class="Bool (strict)"() -> ("Value"=w919:bool)  [unwired: 2 in, 2 out]
                          n397 = Not(x=w919) -> (.not. x?=w918:bool)
                          n398 = property on="PULSE" class="Bool (strict)"("Val(Sgnl)"=w918) -> ()  [unwired: 2 in, 2 out]
                          n399 = property on="Acquire Data" class="Bool (strict)"("Value"=w918) -> ()  [unwired: 2 in, 2 out]
                        }
                      }
                    }
                  }
                }
              }
            }
            n400 = while {
              tunnel: [w936] -> w404
              tunnel: w395 -> [w939]
              tunnel: w396 -> [w922]
              tunnel: w390 -> [w930]
              tunnel: w392 -> [w929]
              tunnel: [w922] -> _
              tunnel: w381 -> [w921]
              tunnel: w380 -> [w920]
              stop <- w936 stop-if-true
              n401 = call "SoftwareGate_Rapid Read.vi"("Timeout (s)"="Timeout (s)", "Channel"="0", "Digitizer Settings"=w921, "AlazarCluster"=w929, "Motion Settings"=w920, "Software Gate"=w930) -> ("gain"=w927:dbl, "Array"=w935:i16[][], "Reverse?"=w934:bool, "error out"=w932:errorcluster)  [unwired: 6 in]
              n402 = case shown="False" w934 {
                tunnel: w935 -> [w941 w942]
                tunnel: [w940 w942] -> w924
                frame False {
                  n403 = call "ReverseData.vi"("Array in"=w941) -> ("Array out"=w940:i16[][])
                }
                frame True {
                }
              }
              n404 = Unbundle By Name(w932) -> ("status"=w931:bool)
              n405 = Wait on Notification(notifier=w939, timeout in ms (-1)=5) -> (timed out?=w937:bool)  [unwired: 2 in, 3 out]
              n406 = Not(x=w937) -> (.not. x?=w936:bool)
              n407 = Bundle("gain"=w927, "status"=FALSE, "Array"=w924, "timeout in ms (-1)"=0, "status"=w931) -> (w926:T45)  [unwired: 1 out]
              n408 = Lossy Enqueue Element(queue=w922, element=w926) -> ()  [unwired: 1 in, 4 out]
            }
            n409 = global read "PulserGlobals.vi" "UTEX VISA"() -> (w374:refnum<visa-resource-name>)
            n410 = call "ReadCurrentSettings.vi"("VISA Refnum in"=w374) -> ("UT340 Controls"=w375:T5)  [unwired: 8 in, 2 out]
            n411 = property on="UT340 Controls" class="Clust (strict)"("Value"=w375) -> ()  [unwired: 2 in, 2 out]
            n412 = Unbundle By Name(w383) -> ("DataBufferQ"=w388:refnum<queue>, "LastNQ"=w387:refnum<queue>, "LastN_JPG_Q"=w386:refnum<queue>)
            n413 = And(x=w404, y=w403) -> (x .and. y?=w397:bool)
            n414 = case shown="True" w397 {
              tunnel: w388 -> [_ w407]
              tunnel: w387 -> [_ w406]
              tunnel: w386 -> [_ w405]
              frame False {
              }
              frame True {
                # "wipe buffers"
                n415 = Flush Queue(queue=w407) -> ()  [unwired: 1 in, 3 out]
                n416 = Flush Queue(queue=w406) -> ()  [unwired: 1 in, 3 out]
                n417 = Flush Queue(queue=w405) -> ()  [unwired: 1 in, 3 out]
              }
            }
          }
          frame #2 {
            n418 = Unbundle By Name(w943) -> ("Main Digitizer"=w944:T15)
            n419 = case shown="\"AlazarTech\"" w944 {
              tunnel: w945 -> [_ _ w952]
              tunnel: w943 -> [_ w946 w949]
              frame "Acqiris Digitizer", Default {
              }
              frame "NI Digitizer" {
                n420 = Unbundle By Name(w946) -> ("Digitizer ID Cluster.NI Instr Handles"=w948:refnum<k15>[])
                n421 = Index Array(array=w948) -> (element=w947:refnum<k15>)  [unwired: 1 in]
                n422 = call <instrlib>:"niScope Abort.vi"("instrument handle"=w947) -> ()  [unwired: 13 in, 2 out]
              }
              frame "AlazarTech" {
                n423 = Unbundle By Name(w949) -> ("Digitizer ID Cluster.Acqiris/Alazar/SP ID"=w951:u32[])
                n424 = Unbundle By Name(w952) -> ("data value reference"=w953:refnum<data-value>)
                n425 = Delete Data Value Reference(data value reference=w953) -> ()  [unwired: 1 in, 2 out]
                n426 = Index Array(array=w951) -> (element=w950:u32)  [unwired: 1 in]
                n427 = call "AlazarAbortAsyncRead.vi"("Handle"=w950) -> ()  [unwired: 1 in, 3 out]
              }
            }
          }
        }
      }
    }
    frame #3 {
      w958 = TRUE ("force destroy? (F)")
      n428 = Unbundle By Name(w957) -> ("DataBufferQ"=w962:refnum<queue>, "LastNQ"=w960:refnum<queue>, "LastN_JPG_Q"=w959:refnum<queue>, "Stop"=w961:refnum<notifier>)
      n429 = Unbundle By Name(w956) -> ("Main Digitizer"=w955:T15)
      n430 = property on="Pulser" class="Enum (strict)"() -> ("Value"=w954:T4)  [unwired: 2 in, 2 out]
      n431 = Release Queue(queue=w959, force destroy? (F)=w958) -> ()  [unwired: 1 in, 3 out]
      n432 = Release Notifier(notifier=w961, force destroy? (F)=w958) -> ()  [unwired: 1 in, 3 out]
      n433 = Release Queue(queue=w962, force destroy? (F)=w958) -> ()  [unwired: 1 in, 3 out]
      n434 = Release Queue(queue=w960, force destroy? (F)=w958) -> ()  [unwired: 1 in, 3 out]
      n435 = case shown="\"UTEX\"" w954 {
        frame Default {
        }
        frame "UTEX" {
          n436 = property on="UT340 Controls" class="Clust (strict)"() -> ("Value"=w966:T5)  [unwired: 2 in, 2 out]
          n437 = Bundle By Name(cluster=w966, "PULSE"=FALSE) -> (w964:T5)
          n438 = call "UTEX Send Values MultiTry.vi"("UT340 Controls"=w964) -> ()  [unwired: 3 in, 2 out]
        }
      }
      n439 = case shown="\"AlazarTech\"" w955 {
        tunnel: w956 -> [_ w969 w975]
        frame "Acqiris Digitizer", Default {
        }
        frame "AlazarTech" {
          n440 = Unbundle By Name(w969) -> ("Digitizer ID Cluster.Acqiris/Alazar/SP ID"=w971:u32[])
          n441 = local write "Acquire Data"(FALSE ("Acquire Data")) -> ()
          n442 = Index Array(array=w971) -> (element=w970:u32)  [unwired: 1 in]
          n443 = call "AlazarConfigureAuxIO.vi"("Parameter"=u32 0, "Mode"=u32 14, "Handle"=w970) -> ()  [unwired: 1 in, 3 out]
        }
        frame "NI Digitizer" {
          n444 = Unbundle By Name(w975) -> ("Digitizer ID Cluster.NI Instr Handles"=w974:refnum<k15>[])
          n445 = Index Array(array=w974) -> (element=w973:refnum<k15>)  [unwired: 1 in]
          n446 = call <instrlib>:"niScope Close.vi"("instrument handle"=w973) -> ()  [unwired: 1 in, 14 out]
        }
      }
      n447 = local write "stop"(FALSE ("stop out")) -> ()
    }
  }
  n448 = global write "DigitizerGlobals.vi" "Digitizer Settings"(w17) -> ()
